vi "Periodic Tasks.vi"(8 "error in":errorcluster) -> ()   [LabVIEW 2012]
doc: "This VI runs in parallel to other tasks. It can contain as many user-defined periodic loops as you need. These can carry out PID or other sorts of timed response."
uses:
  climb_step_state.ctl
  <vilib>/Platform/TimedLoop/XDataNode/timing_clust.ctl
  <vilib>/Platform/TimedLoop/XDataNode/nitl_modes.ctl
  <vilib>/Platform/TimedLoop/XDataNode/wakeup.ctl
  <vilib>/Rock Robotics/WPI/Relay/WPI_RelayValue.ctl
  <vilib>/Rock Robotics/SystemInterfaces/Utilities/FPGA_UtilitiesLED Source.ctl
  <vilib>/Rock Robotics/SystemInterfaces/Utilities/FPGA_UtilitiesLED State.ctl
  Robot Global Data.vi
  <vilib>/Utility/file.llb/Read From Spreadsheet File (string).vi
  <vilib>/Rock Robotics/WPI/RobotDrive/WPI_RobotDriveGetSetRefNum.vi
  <vilib>/platform/TimedLoop/XDataNode/XDataNode.xnode
  <vilib>/Rock Robotics/WPI/Solenoid/WPI_SolenoidSetEnum.vi
  <vilib>/Rock Robotics/WPI/Solenoid/WPI_SolenoidValue.ctl
  <vilib>/Platform/TimedLoop/XDataNode/XDNodeRunTimeDep.lvlib
panel:
  in  "Reset 2":bool
  out "# elements in queue 3":i32
  in  "Reset":bool
  in  "Hold":bool=TRUE
  out "gear":i32
  out "arrived":bool
  in  "Set Point":dbl(slide)=1300.0 scale=-2000.0..1800.0
  in  "Velocity Profile":dbl[][](array[numeric])=[[400.0, 0.23, 0.1], [1000.0, 0.5, 0.1], [0.0, 0.8, 0.2]]
  out "motor":cluster{"Motor":dbl, "gear":i32}(graph)
  out "val":dbl
  out "Rate":cluster{"Rate":dbl, "Distance":dbl}(graph)
  in  "enc ms to wait":u32=100
  in  "Break Engaged 2":i32=120
  in  "Motor Run Time 2":dbl=0.4
  in  "Motor Pwr 2":dbl=-0.1
  in  "Break Disengaged 2":i32
  in  "Delay for disengage 2":dbl=0.2
  out "Enum 2":enum16{"Engaged", "Untension", "Disengaged"}(ring)
  out "Distance 2":dbl
  in  "Output 2":dbl(knob) scale=-1.0..1.0
  in  "Distance desired to\nretract tail hook completely 3":dbl
  in  "Current sensor load 3":dbl
  in  "Distance desired to \nretract (enough to detect if\nwe have weight on current sensor\nin next case) 3":dbl
  in  "distance to extend 3":dbl=850.0
  in  "half extend distance 2":dbl
  out "Rung counter 3":i32
  out "Climb Started? 2":bool
  in  "distance to flip 2":dbl=-600.0
  in  "Auto Flip Speed 2":dbl=-0.18
  out "Climb mode 2":enum16{"Wait", "Automatic", "Manual", "Abort"}(ring)
  out "Climb Step 2":T1
  in  "Climb Extend Tail Speed 2":dbl=1.0
  in  "Climb Retract Tail Speed 2":dbl=-0.9
  in  "Man Flip Speed 2":dbl=-0.75
  out "Turret Home Adjust 2":dbl
  in  "Sky Home Position 2":dbl
  out "Disciplined Sky Enc 2":dbl
  out "Sky Enc 2":dbl
  in  "Slow Retract 2":dbl=-0.25
  in  "Slow Extend 2":dbl=0.25
  in  "Robot Detect":T2(radio)
  out "Robot Detect":i32
  out "MAC Address":string
  out "Personality":string
  in  "Tab Control":T3(tab)
  out "FIFO":u32(graph)
  out "Shot Profile":dbl(graph)=3763.879304936955
  in  "Count":i32=80
  out "RPM @ Shot":dbl
  out "% err":dbl
  in  "Fire Log Enable":bool=TRUE
  in  "loop period (ms)":u32=200
  out "iterations":i32
  out "FIFO elements":u32
  in  "Burst":i32=75
  out "Save":bool
  out "Left Wheel Encoder":dbl
  out "Right Wheel Encoder":dbl
  out "LStopped":bool
  out "RStopped":bool
  out "Motor":dbl(graph)
  in  "Position":dbl(knob) scale=0.0..1500.0
  in  "SkyHook":dbl(knob) scale=-1.0..1.0
  out "Distance":dbl
  out "Home":bool
  in  "Motor Coerce":dbl=0.9
  in  "Lo Limit":dbl
  in  "Hi Limit":dbl=1500.0
  out "At Lo":bool
  out "At Hi":bool
  in  "Near Limit":dbl=200.0
  in  "Speed near Lim Up":dbl=0.2
  in  "Period":i64=51
  in  "Speed near Lim Dn":dbl=0.1
  in  "PID":bool
  in  "P":dbl(knob) scale=0.0..0.01
  out "err":dbl
  out "Rate":dbl
  in  "Auto Pitch":bool=TRUE
  in  "Elev Stable Tol (sec)":dbl(knob)=0.5044674819294696 scale=0.0..1.0
  out "Q 2":i32(graph)
  out "Current":dbl(graph)
  in  "A / V":dbl=13.66
  in  "Sample (s)":dbl=0.1
  in  "Log Enable":bool
  out "# elements in queue 2":i32
  out "Compressor Running":bool
  out "Right Odometer":dbl
  out "Left Odometer":dbl
  in  "Sample Rate (sec)":dbl=0.5
  in  "Sample?":bool=TRUE
  in  "Sample Rate (sec) 2":dbl=0.1
  in  "General Log Enable":bool=TRUE
  out "# elements in queue":i32
  in  "Gyro Gain (VoltsPerDegree/Second)":dbl(knob)=0.006611706614844206 scale=0.0..0.01
  out "Angle":dbl
  out "CornerShot Pitch":dbl
  out "Tow3 Offset Pitch":dbl
  out "Tow3 Offset RPM":dbl
  out "Tow1 Offset RPM":dbl
  out "Tow2 Offset RPM":dbl
  out "Tow1 Offset Pitch":dbl
  out "Tow2 Offset Pitch":dbl
  out "Std RPM":dbl
  out "Std Pitch":dbl
  out "Auton RPM":dbl
  out "Auton Pitch":dbl
  out "Wing RPM":dbl
  out "Wing Pitch":dbl
  out "Parameter Read":i32
  out "Tow1 Offset RPM 2":dbl
  out "Tow1 Offset Pitch 2":dbl
  out "Tow2 Offset RPM 2":dbl
  out "Tow2 Offset Pitch 2":dbl
  out "Tow3 Offset RPM 2":dbl
  out "Tow3 Offset Pitch 2":dbl
  out "QC iter":i32
  out "FIFO Elements":u32(graph)
  in  "loop period (ms) 2":u32=200
  out "Save Ascent":bool
  in  "Auto Ascent Log Enable":bool
  # "TDMS"
  # "TDMS"
  # "TDMS"
  # "TDMS"
  # "Range"
  # "Rate"
  # "Accel"
  # "Fire Cntrl Loop"
  # "Fire Cntrl Logging Loop"
  # "Sensor sensitivity is 73.20 mV / Amp"
  # "which is: 13.66 Amps / Volt"
  # "TDMS"
  # "Off will Disable\nOn will Sample at Rate"
  # "TDMS"
  # "On will sample at Rate\nOff will Disable"
  # "Positive Angles result from CW turns\nlooking down on Robot"
  # "Pos values back up\nNeg values go forward"
  # "Tower Shots"
  # "Auto Ascent Log"
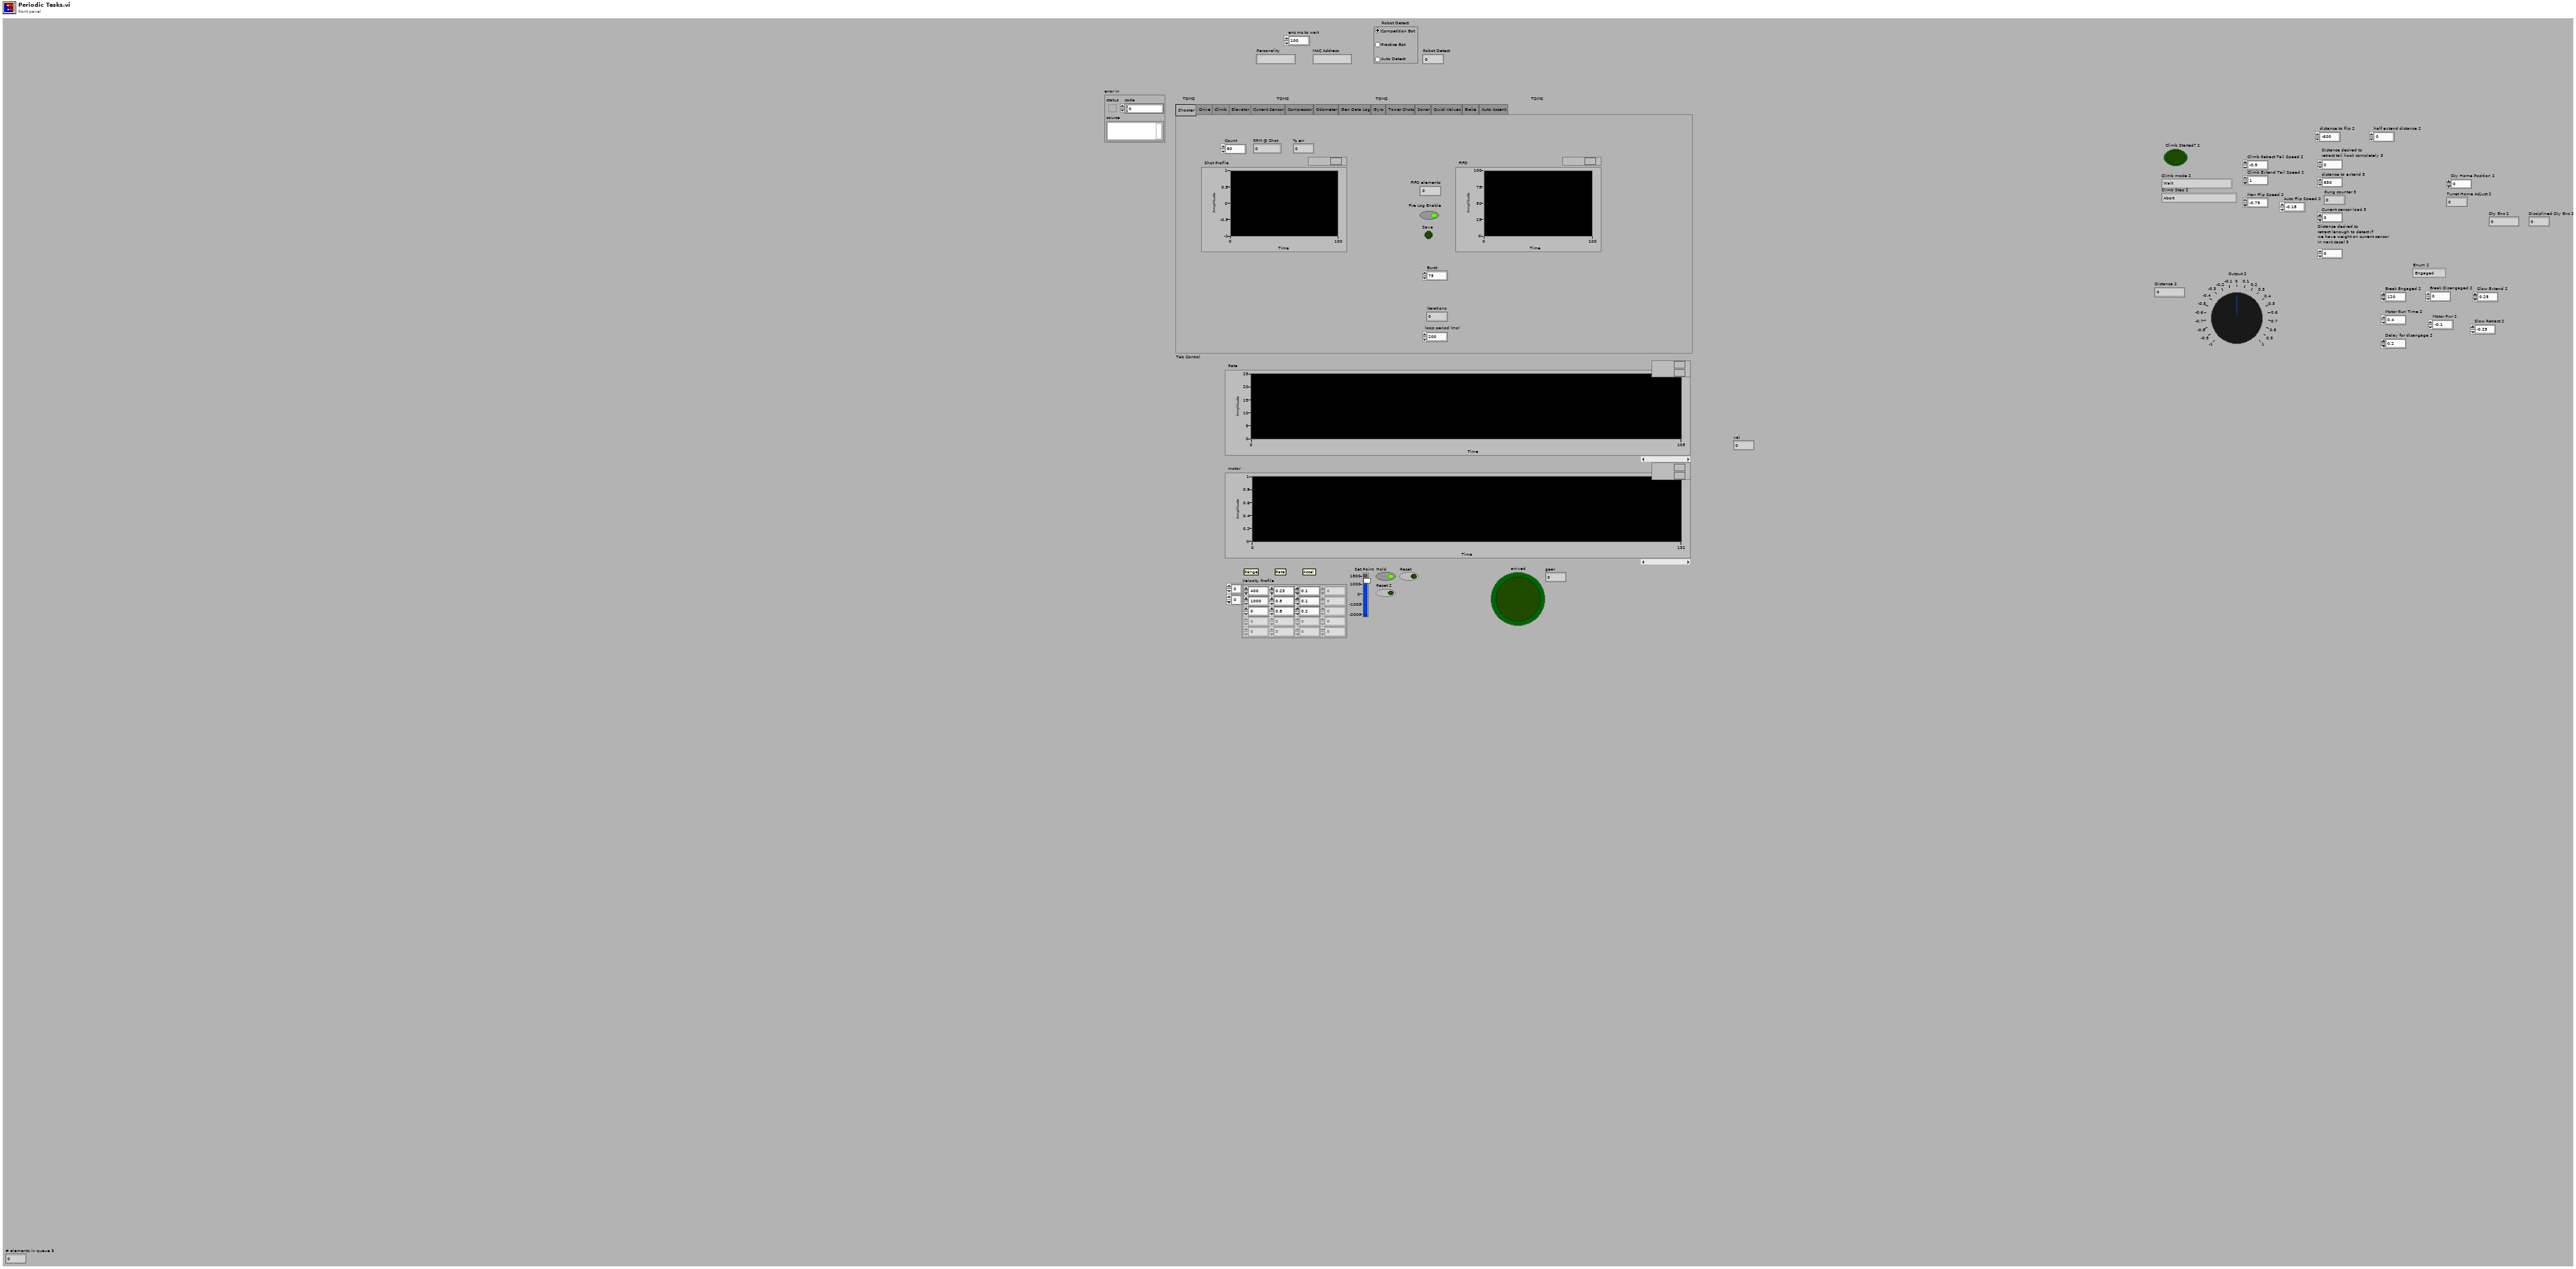
[diagram p1: front panel]
types:
  T1 = typedef "climb_step_state.ctl" = enum16{"Abort", "Approach Bar", "Approach +", "Climb Step 1", "Climb Step 2", "Climb Step 3", "Climb Step 4", "Climb Step 5", "Climb Step 6", "Climb Step 7", "Check Finished", "Check Continue"}
  T2 = enum32{"Competition Bot", "Practice Bot", "Auto Detect"}
  T3 = enum32{"Shooter", "Drive", "Climb", "Elevator", "Current Sensor", "Compressor", "Odometer", "Gen Data Log", "Gyro", "Tower Shots", "Sonar", "Quick Values", "Brake", "Auto Ascent"}
  T4 = enum16{"open", "open or create", "create or replace", "create", "open (read-only)"}
  T5 = cluster{"Driver Station Digital Input (1-8)[0]":bool, "Driver Station Digital Input (1-8)[1]":bool, "Driver Station Digital Input (1-8)[2]":bool, "Driver Station Digital Input (1-8)[3]":bool, "Driver Station Digital Input (1-8)[4]":bool, "Driver Station Digital Input (1-8)[5]":bool, "Driver Station Digital Input (1-8)[6]":bool, "Driver Station Digital Input (1-8)[7]":bool, "Driver Station Digital Input (1-8)[8]":bool}
  T6 = typedef "WPI_CounterDevRef.ctl" = cluster{"DevStatus":errorcluster, "CntIndex":T7}
  T7 = typedef "FPGA_CounterCtrSystemIndex.ctl" = enum8{"Ctr 0", "Ctr 1", "Ctr 2", "Ctr 3", "Ctr 4", "Ctr 5", "Ctr 6", "Ctr 7", "Invalid"}
  T8 = typedef "WPI_MotorControlDeviceRef.ctl" = cluster{"DeviceStatus":errorcluster, "Type":enum16{"PWM", "CAN"}, "PWM":cluster{"Digital Module":T9, "PWM Channel":T10, "DeadBand":T11}, "CAN":cluster{"Device Number":u8, "Control Mode":T12, "Semaphore":T13, "Max Vout":dbl}, "Invert":bool, "TransformRef":T14, "InvTransformRef":T14}
  T9 = typedef "FPGA_TypedefDigitalModule.ctl" = enum16{"Digital Module 1", "Digital Module 2"}
  T10 = typedef "FPGA_DIOPWMChannel.ctl" = enum8{"PWM 1", "PWM 2", "PWM 3", "PWM 4", "PWM 5", "PWM 6", "PWM 7", "PWM 8", "PWM 9", "PWM 10", "Invalid"}
  T11 = typedef "WPI_PWMDeadband.ctl" = cluster{"Name":string, "maxPositivePwm":i32, "minPositivePwm":i32, "centerPwm":i32, "maxNegativePwm":i32, "minNegativePwm":i32, "angularRange":u16}
  T12 = typedef "WPI_CANJaguar_ControlMode.ctl" = enum8{"Percent VBus", "Current", "Speed", "Position", "Voltage"}
  T13 = typedef "Semaphore RefNum" = refnum<k1>
  T14 = typedef "WPI_PWMTransform_ConPane.ctl" = refnum<vi>
  T15 = typedef "WPI_GyroDevRef.ctl" = cluster{"DevStatus":errorcluster, "Analog Module":T16, "Analog Channel":T17, "Offset":dbl, "Gain (VoltsPerDegree/Second)":dbl}
  T16 = typedef "FPGA_TypedefAnalogModule.ctl" = enum16{"Analog Module 1", "Analog Module 2"}
  T17 = typedef "FPGA_AIChannel.ctl" = enum8{"AI 1", "AI 2", "AI 3", "AI 4", "AI 5", "AI 6", "AI 7", "AI 8", "Invalid"}
  T18 = typedef "WPI_EncoderDevRef.ctl" = cluster{"DevStatus":errorcluster, "EncoderIndex":T19, "CounterIndex":T7, "DistancePerCount":dbl, "Decoding Type":T20}
  T19 = typedef "FPGA_EncoderIdx.ctl" = enum8{"Enc 0", "Enc 1", "Enc 2", "Enc 3", "Invalid"}
  T20 = typedef "WPI_EncoderType.ctl" = enum16{"1x", "2x", "4x"}
  T21 = typedef "WPI_SolenoidDevRef.ctl" = cluster{"DevStatus":errorcluster, "Solenoid Module":T22, "Forward Solenoid Channel":T23, "Reverse Solenoid Channel":T23}
  T22 = typedef "FPGA_TypedefSolenoidModule.ctl" = enum16{"Solenoid Module 1", "Solenoid Module 2"}
  T23 = typedef "WPI_SolenoidChannel.ctl" = enum8{"Solenoid 1", "Solenoid 2", "Solenoid 3", "Solenoid 4", "Solenoid 5", "Solenoid 6", "Solenoid 7", "Solenoid 8", "Invalid"}
  T24 = typedef "WPI_RelayDevRef.ctl" = cluster{"DevStatus":errorcluster, "Relay Channel":T25, "Digital Module":T9, "Relay Direction":T26}
  T25 = typedef "FPGA_DIORelayChannel.ctl" = enum8{"Relay 1", "Relay 2", "Relay 3", "Relay 4", "Relay 5", "Relay 6", "Relay 7", "Relay 8", "Invalid"}
  T26 = typedef "WPI_RelayDirection.ctl" = enum16{"Both directions", "Forward only", "Reverse only"}
  T27 = typedef "WPI_DigitalInputDevRef.ctl" = cluster{"DevStatus":errorcluster, "DIO Channel":T28, "Digital Module":T9}
  T28 = typedef "FPGA_DIOChannel.ctl" = enum8{"DIO 1", "DIO 2", "DIO 3", "DIO 4", "DIO 5", "DIO 6", "DIO 7", "DIO 8", "DIO 9", "DIO 10", "DIO 11", "DIO 12", "DIO 13", "DIO 14", "Invalid"}
  T29 = typedef "XDNodeRunTimeDep.lvlib/timing_clust.ctl" = cluster{"Expected End [f-1]":u64, "Actual End [f-1]":u64, "Finished Late? [f-1]":bool, "Expected End [i-1]":u64, "Actual End [i-1]":u64, "Finished Late? [i-1]":bool, "Expected Start [i]":u64, "Actual Start [i]":u64, "Expected Start [f]":u64, "Actual Start [f]":u64, "Source Name":string, "Structure Name":string, "Period":i64, "Deadline":i64, "Offset":i64, "Start":i64, "Priority":i32, "Timeout":i32, "Mode":T30, "Wakeup Reason":T31, "Error":errorcluster, "Source Type":string, "Secondary Source Type":string, "Global End Time":u64, "Global Start Time":u64, "Frame Duration":u64, "Iteration Duration":u64, "Assigned CPU":i32, "I/O Scan Engine Mode":u32}
  T30 = typedef "XDNodeRunTimeDep.lvlib/nitl_modes.ctl" = enum32{"No Change", "Process missed periods, maintain original phase", "Discard missed periods, maintain original phase", "Process missed periods, ignore original phase", "Discard missed periods, ignore original phase"}
  T31 = typedef "XDNodeRunTimeDep.lvlib/wakeup.ctl" = enum32{"Normal", "Aborted", "Asynchronous wakeup", "Timing source error", "Timed loop error", "Timeout"}
  T32 = typedef "WPI_AnalogChannelDevRef.ctl" = cluster{"DevStatus":errorcluster, "Analog Module":T16, "Analog Channel":T17}
  T33 = typedef "FPGA_UtilitiesLED State.ctl" = enum16{"Off", "On", "Toggle"}
  T34 = typedef "FPGA_UtilitiesLED Source.ctl" = enum16{"User LED", "FPGA LED"}
  T35 = cluster{"all rows[0]":string, "all rows[1]":string, "all rows[2]":string, "all rows[3]":string, "all rows[4]":string, "all rows[5]":string, "all rows[6]":string, "all rows[7]":string, "all rows[8]":string}
  T36 = typedef "fire_step_state.ctl" = enum16{"static", "manual", "saftey_down", "saftey_up", "check_saftey", "fire"}
  T37 = typedef "WPI_RelayValue.ctl" = enum16{"Off", "On", "Forward", "Reverse"}
  T38 = typedef "WPI_ServoDeviceRef.ctl" = cluster{"DeviceStatus":errorcluster, "Digital Module":T9, "PWM Channel":T10, "DeadBand":T11}
  T39 = typedef "WPI_RobotDriveDevRef.ctl" = cluster{"DevStatus":errorcluster, "Motors[]":T8[], "Square Inputs":bool, "Max Output":dbl, "Isochronous":bool}
  T40 = typedef "WPI_SolenoidValue.ctl" = enum16{"Off", "On", "Forward", "Reverse"}
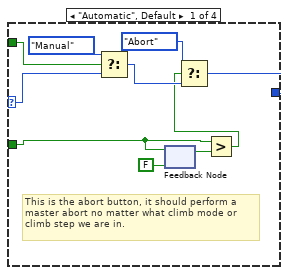
[diagram p2: hidden frame]
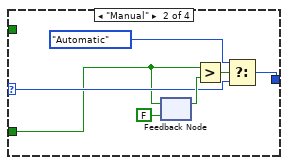
[diagram p3: hidden frame]
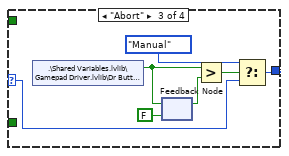
[diagram p4: hidden frame]
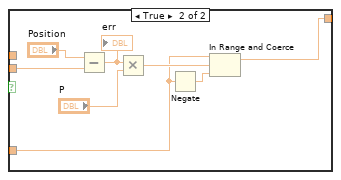
[diagram p5: hidden frame]
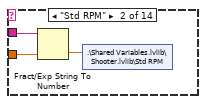
[diagram p20: hidden frame]
diagram:
  w6 = 5 ("dimension size")
  w13 = climb_step_state."Approach Bar" ("Climb Step")
  w65 = path "C:/tmp/Odometer.tdms" ("file path (dialog if empty)")
  (unwired) "NI_DiskCacheSize"
  w114 = 18 ("dimension size")
  (unwired) "This code flashes the USER1 LED on the cRIO.  It is a simple way to let you know your code is running on the cRIO.  You can leave this code if you find it helpful, or delete it if you don't want it."
  (unwired) "This VI is a good place to take care of periodic tasks such as control loops.\n\nAdd code to the existing loops, or duplicate a loop to define a new rate. You can allocate I/O references here, or in Begin.vi.\n\nPeriodic loops will often operate with setpoints from other loops. Use a global variable such as Robot Global Data for sharing data between loops."
  # "Auto Ascent FIFO Setup"
  # "Size of Auto Ascent Log"
  # "Periodic Data FIFO Setup"
  # "Odometer"
  # "Size of Fire Cntrl Log"
  # "Pre-Allocate Array to improve \nDeterminism when Data Logging"
  # "Removed Safety Servo and States\nBatWings\nDisc Drive is full time\nRemoved Override\nRemoved Drive stopped\nRemoved settings for other shooter\nTrimmed Log entries"
  # "Data Log Enable"
  # "Periodic Data Log Setup"
  n1 = while {
    stop <- FALSE stop-if-true
    n2 = call <vilib>:"WPI_DriverStationGet Digital Input.vi"() -> ("Driver Station Digital Input (1-8)"=w136:bool[])  [unwired: 11 in]
    n3 = Array To Cluster(array=w136) -> (cluster=w135:T5)
    n4 = Unbundle By Name(w135) -> ("Driver Station Digital Input (1-8)[7]"=w134:bool)
    n5 = Wait (ms)(milliseconds to wait=u32 500) -> ()  [unwired: 1 out]
    n6 = shared-variable ".\\Shared Variables.lvlib\\System.lvlib\\Data Log"(w134) -> ()  [unwired: 1 in, 1 out]
  }
  n7 = Get Date/Time In Seconds() -> (seconds since 1Jan1904=w124:timestamp)
  n8 = Format Date/Time String(time format string (%c)="%m-%#d-%Y %H%M", seconds (now)=w124, UTC format=FALSE) -> (date/time string=w129:string)
  n9 = Concatenate Strings("PeriodicDataLog" ("string"), w129, ".tdms" ("string")) -> (w131:string)
  n10 = Build Path(base path=path "C:/tmp" ("file path (dialog if empty)"), name or relative path=w131) -> (appended path=w111:path)
  n11 = TDMS Open(6:TRUE ("disable buffering? (T)"), 7:enum16{"1.0", "2.0"}."2.0" ("file format version (2.0)"), 10:T4."open or create" ("operation (0:open)"), 11:w111) -> (3:w93:refnum<k34>)  [unwired: 2 in, 1 out]
  n12 = for {
    N: 18 -> [_]
    tunnel: string[] ["Time", "Iteration", "Mode", "Raw Prime", "Cultured Prime", "Raw On Deck", "Cultured On Deck", "Button 6 Op (Fire)", "Fire Case", "RPM", "Elevator", "Shooter Bump", "Elevator Bump", "Button 2 Op (Wish)", "Shooter Stable", "Indexer", "Air Lock", "FIFO Buffer", "", "", "", "", "", "", "", "", ""] ("channel name(s) in (Untitled)") -> [w144] mode=indexing
    tunnel: "Fire Control" ("group name in (Untitled)") -> [w143]
    tunnel: w93 -> [w142]
    tunnel: [w141] -> w34
    tunnel: "NI_MimimumBufferSize" -> [w140]
    tunnel: 1000 -> [w139]
    n13 = TDMS Set Properties(5:w139, 7:w140, 9:w144, 10:w143, 11:w142) -> (3:w141:refnum<k34>)  [unwired: 1 in, 3 out]
  }
  n14 = Initialize Array(0 ("element"), w6) -> (w18:i32[])
  n15 = Initialize Array(0 ("element"), w114) -> (w112:i32[])
  n16 = To Unsigned Long Integer(number=w6) -> (unsigned 32bit integer=w5:u32)
  n17 = To Unsigned Long Integer(number=w114) -> (unsigned 32bit integer=w113:u32)
  n18 = RT FIFO Create(0:"Auto Ascent FIFO" ("name (unnamed)"), 1:w18, 4:u32 100 ("size (10)"), 6:w5) -> (8:w19:refnum<k33>)  [unwired: 4 in, 2 out]
  n19 = RT FIFO Create(0:"Fire Control FIFO" ("name (unnamed)"), 1:w112, 4:u32 100 ("size (10)"), 6:w113) -> (8:w116:refnum<k33>)  [unwired: 4 in, 2 out]
  n20 = call "cRIO MAC.vi"() -> ("MAC Address"=→"MAC Address":string, "Personality"=w96:string)  [unwired: 2 in]
  "Personality" <- w96
  n21 = call <vilib>:"WPI_CounterRefNum Registry Get.vi"("refnum name"="shooterRpm") -> ("CounterDevRef"=w86:T6)  [unwired: 9 in, 1 out]
  n22 = call <vilib>:"WPI_MotorControlRefNum Registry Get.vi"("refnum name"="shooterThrust") -> ("MotorControlDevRef"=w84:T8)  [unwired: 9 in, 1 out]
  n23 = disable-structure shown="Disabled" {
    disable-tunnel: w65 -> [w145 _]
    frame Disabled {
      n24 = TDMS Defragment(7:w145) -> ()  [unwired: 1 in, 1 out]
    }
    frame Enabled {
    }
  }
  n25 = Get Date/Time In Seconds() -> (seconds since 1Jan1904=w56:timestamp)
  n26 = Initialize Array(0.0 ("element"), 3 ("dimension size")) -> (w47:dbl[])
  n27 = call <vilib>:"WPI_GyroRefNum Registry Get.vi"("refnum name"="turnGyro") -> ("GyroDevRef"=w70:T15)  [unwired: 9 in, 1 out]
  n28 = TDMS Open(7:enum16{"1.0", "2.0"}."2.0" ("file format version (2.0)"), 10:T4."open or create" ("operation (0:open)"), 11:w65) -> (3:w33:refnum<k34>)  [unwired: 3 in, 1 out]
  n29 = call <vilib>:"WPI_EncoderRefNum Registry Get.vi"("refnum name"="leftWheelEncoder") -> ("EncoderDevRef"=w74:T18)  [unwired: 9 in, 1 out]
  n30 = call <vilib>:"WPI_EncoderRefNum Registry Get.vi"("refnum name"="rightWheelEncoder") -> ("EncoderDevRef"=w73:T18)  [unwired: 9 in, 1 out]
  n31 = Initialize Array(0.0 ("element"), 4 ("dimension size")) -> (w39:dbl[])
  n32 = call <vilib>:"WPI_SolenoidRefNum Registry Get.vi"("refnum name"="discSolenoid") -> ("SolenoidDevRef"=w101:T21)  [unwired: 9 in, 1 out]
  n33 = call <vilib>:"WPI_RelayRefNum Registry Get.vi"("refnum name"="conveyor") -> ("RelayDevRef"=w99:T24)  [unwired: 9 in, 1 out]
  n34 = call <vilib>:"WPI_SolenoidRefNum Registry Get.vi"("refnum name"="fireSolenoid") -> ("SolenoidDevRef"=w100:T21)  [unwired: 9 in, 1 out]
  n35 = call <vilib>:"WPI_DigitalInputRefNum Registry Get.vi"("refnum name"="breakBeamOnDeck") -> ("DigitalInputDevRef"=w102:T27)  [unwired: 9 in, 1 out]
  n36 = call <vilib>:"WPI_DigitalInputRefNum Registry Get.vi"("refnum name"="breakBeamPrime") -> ("DigitalInputDevRef"=w103:T27)  [unwired: 9 in, 1 out]
  n37 = To Double Precision Float(number=w56) -> (double precision float=w55:dbl)
  n38 = call <vilib>:"WPI_DigitalInputRefNum Registry Get.vi"("refnum name"="compressorSwitch") -> ("DigitalInputDevRef"=w132:T27)  [unwired: 9 in, 1 out]
  n39 = node-c288(i64 51 ("Period")) -> (w30:T29)  [unwired: 3 in]
  n40 = node-c288(i64 16 ("Period")) -> (w110:T29)  [unwired: 3 in]
  n41 = node-c288(i64 11 ("Period")) -> (w89:T29)  [unwired: 3 in]
  n42 = Get Date/Time In Seconds() -> (seconds since 1Jan1904=w44:timestamp)
  n43 = Get Date/Time In Seconds() -> (seconds since 1Jan1904=w52:timestamp)
  n44 = Obtain Queue(max queue size (-1, unlimited)=100, name (unnamed)="Q", element data type=w47) -> (queue out=w46:refnum<queue>)  [unwired: 2 in, 2 out]
  n45 = Obtain Queue(max queue size (-1, unlimited)=100, name (unnamed)="Q2", element data type=w39) -> (queue out=w38:refnum<queue>)  [unwired: 2 in, 2 out]
  n46 = call <vilib>:"WPI_AnalogChannelRefNum Registry Get.vi"("refnum name"="climbMotorCurrent") -> ("AIDeviceRef"=w35:T32)  [unwired: 9 in, 1 out]
  n47 = To Double Precision Float(number=w44) -> (double precision float=w43:dbl)
  n48 = To Double Precision Float(number=w52) -> (double precision float=w51:dbl)
  n49 = while {
    stop <- FALSE stop-if-true
    # "This global is written to in the Autonomous and Teleop VIs"
    # "Flash the USER1 LED with the rate controlled from Autonomous and Teleop"
    n50 = global read "Robot Global Data.vi" "LED toggle rate (ms)"() -> (w146:u32)
    n51 = call <vilib>:"WPI_UtilitiesFRC LEDs.vi"("State"=FPGA_UtilitiesLED_State."Toggle", "LED Type"=FPGA_UtilitiesLED_Source."User LED") -> ()  [unwired: 1 in, 9 out]
    n52 = Wait (ms)(milliseconds to wait=w146) -> ()  [unwired: 1 out]
  }
  n53 = while "Robot Detect Loop" {
    tunnel: w96 -> [w152]
    tunnel: [w150] -> w119
    i -> [w153]
    stop <- w156 stop-if-true
    # "Auto-Detect"
    n54 = Equal?(x="Robot Detect", y=T2."Competition Bot") -> (x = y?=w158:bool)
    n55 = Equal?(x="Robot Detect", y=T2."Practice Bot") -> (x = y?=w157:bool)
    n56 = Select(t="Pract Bot - Friz 1", s=w157, f=w152) -> (s? t:f=w159:string)
    n57 = Not Equal?(x=w152, y="") -> (x != y?=w154:bool)
    n58 = Select(t="Comp Bot - Friz 2", s=w158, f=w159) -> (s? t:f=w150:string)
    n59 = global write "Robot Global Data.vi" "Personality"(w150) -> ()
    n60 = Compound Arithmetic op=OR(w158, w157, w154) -> (w156:bool)
    n61 = Wait (ms)(milliseconds to wait=u32 30) -> ()  [unwired: 1 out]
    "Robot Detect" <- w153
  }
  n62 = while "Quick-change parameters" {
    tunnel: [w165] -> w95
    stop <- w165 stop-if-true
    w165 = TRUE
    n63 = call-poly <vilib>:"Read From Spreadsheet File.vi"("delimiter (\\t)"="=" ("delimiter (\\t)"), "file path (dialog if empty)"=path "C:/tmp/2013 Code Parameters.csv" ("datalog path (use dialog)")) -> ("all rows"=w166:string[][])  [unwired: 5 in, 4 out]
    n64 = for {
      tunnel: w166 -> [w174] mode=indexing
      i -> [w169]
      n65 = Array To Cluster(array=w174) -> (cluster=w173:T35)
      n66 = Unbundle By Name(w173) -> ("all rows[0]"=w172:string, "all rows[1]"=w171:string)
      n67 = case shown="\"Auton RPM\"" w172 {
        tunnel: w171 -> [_ w177 w180 w183 w186 w189 w192 w195 w198 w201 w204 w207 w210 w213]
        tunnel: 0.0 -> [_ w176 w179 w182 w185 w188 w191 w194 w197 w200 w203 w206 w209 w212]
        frame "", Default {
        }
        frame "Std RPM" {
          n68 = Fract/Exp String To Number(string=w177, default (0 dbl)=w176) -> (number=w175:dbl)  [unwired: 2 in, 1 out]
          n69 = shared-variable ".\\Shared Variables.lvlib\\Shooter.lvlib\\Std RPM"(w175) -> ()  [unwired: 1 in, 1 out]
        }
        frame "Std Pitch" {
          n70 = Fract/Exp String To Number(string=w180, default (0 dbl)=w179) -> (number=w178:dbl)  [unwired: 2 in, 1 out]
          n71 = shared-variable ".\\Shared Variables.lvlib\\Elevator.lvlib\\Std Pitch"(w178) -> ()  [unwired: 1 in, 1 out]
        }
        frame "Auton RPM" {
          n72 = Fract/Exp String To Number(string=w183, default (0 dbl)=w182) -> (number=w181:dbl)  [unwired: 2 in, 1 out]
          n73 = shared-variable ".\\Shared Variables.lvlib\\Shooter.lvlib\\Auton RPM"(w181) -> ()  [unwired: 1 in, 1 out]
        }
        frame "Auton Pitch" {
          n74 = Fract/Exp String To Number(string=w186, default (0 dbl)=w185) -> (number=w184:dbl)  [unwired: 2 in, 1 out]
          n75 = shared-variable ".\\Shared Variables.lvlib\\Elevator.lvlib\\Auton Pitch"(w184) -> ()  [unwired: 1 in, 1 out]
        }
        frame "Wing RPM" {
          n76 = Fract/Exp String To Number(string=w189, default (0 dbl)=w188) -> (number=w187:dbl)  [unwired: 2 in, 1 out]
          n77 = shared-variable ".\\Shared Variables.lvlib\\Shooter.lvlib\\Wing RPM"(w187) -> ()  [unwired: 1 in, 1 out]
        }
        frame "Wing Pitch" {
          n78 = Fract/Exp String To Number(string=w192, default (0 dbl)=w191) -> (number=w190:dbl)  [unwired: 2 in, 1 out]
          n79 = shared-variable ".\\Shared Variables.lvlib\\Elevator.lvlib\\Wing Pitch"(w190) -> ()  [unwired: 1 in, 1 out]
        }
        frame "Tow1 Offset RPM" {
          n80 = Fract/Exp String To Number(string=w195, default (0 dbl)=w194) -> (number=w193:dbl)  [unwired: 2 in, 1 out]
          "Tow1 Offset RPM" <- w193
          n81 = shared-variable ".\\Shared Variables.lvlib\\Shooter.lvlib\\Tow1 Offset RPM"(w193) -> ()  [unwired: 1 in, 1 out]
        }
        frame "Tow1 Offset Pitch" {
          n82 = Fract/Exp String To Number(string=w198, default (0 dbl)=w197) -> (number=w196:dbl)  [unwired: 2 in, 1 out]
          "Tow1 Offset Pitch" <- w196
          n83 = shared-variable ".\\Shared Variables.lvlib\\Elevator.lvlib\\Tow1 Offset Pitch"(w196) -> ()  [unwired: 1 in, 1 out]
        }
        frame "Tow2 Offset RPM" {
          n84 = Fract/Exp String To Number(string=w201, default (0 dbl)=w200) -> (number=w199:dbl)  [unwired: 2 in, 1 out]
          "Tow2 Offset RPM" <- w199
          n85 = shared-variable ".\\Shared Variables.lvlib\\Shooter.lvlib\\Tow2 Offset RPM"(w199) -> ()  [unwired: 1 in, 1 out]
        }
        frame "Tow2 Offset Pitch" {
          n86 = Fract/Exp String To Number(string=w204, default (0 dbl)=w203) -> (number=w202:dbl)  [unwired: 2 in, 1 out]
          "Tow2 Offset Pitch" <- w202
          n87 = shared-variable ".\\Shared Variables.lvlib\\Elevator.lvlib\\Tow2 Offset Pitch"(w202) -> ()  [unwired: 1 in, 1 out]
        }
        frame "Tow3 Offset RPM" {
          n88 = Fract/Exp String To Number(string=w207, default (0 dbl)=w206) -> (number=w205:dbl)  [unwired: 2 in, 1 out]
          "Tow3 Offset RPM" <- w205
          n89 = shared-variable ".\\Shared Variables.lvlib\\Shooter.lvlib\\Tow3 Offset RPM"(w205) -> ()  [unwired: 1 in, 1 out]
        }
        frame "Tow3 Offset Pitch" {
          n90 = Fract/Exp String To Number(string=w210, default (0 dbl)=w209) -> (number=w208:dbl)  [unwired: 2 in, 1 out]
          "Tow3 Offset Pitch" <- w208
          n91 = shared-variable ".\\Shared Variables.lvlib\\Elevator.lvlib\\Tow3 Offset Pitch"(w208) -> ()  [unwired: 1 in, 1 out]
        }
        frame "CornerShot Pitch" {
          n92 = Fract/Exp String To Number(string=w213, default (0 dbl)=w212) -> (number=w211:dbl)  [unwired: 2 in, 1 out]
          "CornerShot Pitch" <- w211
          n93 = shared-variable ".\\Shared Variables.lvlib\\Elevator.lvlib\\CornerShot Pitch"(w211) -> ()  [unwired: 1 in, 1 out]
        }
      }
      "QC iter" <- w169
    }
  }
  n94 = timed-loop "Fire Control Loop\nTime Critical" {
    tunnel: w103 -> [w218]
    tunnel: w102 -> [w247]
    tunnel: w101 -> [w246]
    tunnel: w100 -> [w245]
    tunnel: w99 -> [w244]
    tunnel: w112 -> [w219]
    timing: w110 -> [_]
    timing-out: [_] -> w109
    tunnel: w116 -> [w223]
    tunnel: w55 -> [w216]
    i -> [w217]
    stop <- FALSE stop-if-true
    w230 = 4200.0 ("x")
    n95 = feedback #1() -> (w225:T36)  [unwired: 1 in]
    n96 = call "Fire Control Loop.vi"("Prime BB DevRef"=w218, "OnDeck BB DevRef"=w247, "Fire Log Enable"="Fire Log Enable", "FireDevRef"=w245, "Time Ref"=w216, "ConveyorDevRef"=w244, "rt fifo"=w223, "Fire State In"=w225, "LogArray"=w219, "iteration"=w217, "IndexerDevRef"=w246) -> ("Fire"=w236:bool, "Fire State Out"=w226:T36, "# elements"=w222:u32)  [unwired: 2 in]
    "FIFO elements" <- w222
    "FIFO" <- w222
    n97 = feedback-in #1(w226) -> ()
    n98 = shared-variable ".\\Shared Variables.lvlib\\Shooter.lvlib\\Shooter RPM Response"() -> (w234:dbl)  [unwired: 1 in, 1 out]
    n99 = local read "Burst"() -> (w221:i32)
    n100 = Greater?(x=w222, y=w221) -> (0:→"Save":bool)
    n101 = feedback #2() -> (w235:bool)  [unwired: 1 in]
    n102 = feedback-in #2(w236) -> ()
    n103 = Greater?(x=w236, y=w235) -> (0:w233:bool)
    n104 = feedback #3(0) -> (w242:i32)
    n105 = Select(t=w217, s=w233, f=w242) -> (s? t:f=w241:i32)
    n106 = feedback-in #3(w241) -> ()
    n107 = feedback #4() -> (w237:dbl)  [unwired: 1 in]
    n108 = Select(t=w234, s=w233, f=w237) -> (s? t:f=w232:dbl)
    "RPM @ Shot" <- w232
    n109 = feedback-in #4(w232) -> ()
    n110 = Add(x=w241, y="Count") -> (x+y=w239:i32)
    n111 = Less Or Equal?(x=w217, y=w239) -> (x <= y?=w238:bool)
    n112 = case shown="True" w238 {
      tunnel: w234 -> [_ w248]
      frame False {
      }
      frame True {
        "Shot Profile" <- w248
      }
    }
    n113 = Subtract(x=w230, y=w232) -> (x-y=w231:dbl)
    n114 = Divide(x=w231, y=w230) -> (x/y=w229:dbl)
    n115 = Multiply(x=w229, y=100.0) -> (x*y=→"% err":dbl)
    n116 = call "Elapsed Times.vi"("Call Name"="F") -> ()  [unwired: 2 in, 1 out]
  }
  n117 = while "Quick-change File I/O Verification Display" {
    i -> [w274]
    stop <- w277 stop-if-true
    n118 = shared-variable ".\\Shared Variables.lvlib\\Shooter.lvlib\\Std RPM"() -> (→"Std RPM":dbl, error out=w261:errorcluster)  [unwired: 1 in]
    n119 = shared-variable ".\\Shared Variables.lvlib\\Elevator.lvlib\\Std Pitch"(error in=w261) -> (→"Std Pitch":dbl, error out=w260:errorcluster)
    n120 = shared-variable ".\\Shared Variables.lvlib\\Shooter.lvlib\\Auton RPM"(error in=w260) -> (→"Auton RPM":dbl, error out=w259:errorcluster)
    n121 = shared-variable ".\\Shared Variables.lvlib\\Elevator.lvlib\\Auton Pitch"(error in=w259) -> (→"Auton Pitch":dbl, error out=w258:errorcluster)
    n122 = shared-variable ".\\Shared Variables.lvlib\\Shooter.lvlib\\Wing RPM"(error in=w258) -> (→"Wing RPM":dbl, error out=w257:errorcluster)
    n123 = shared-variable ".\\Shared Variables.lvlib\\Elevator.lvlib\\Wing Pitch"(error in=w257) -> (→"Wing Pitch":dbl, error out=w256:errorcluster)
    n124 = shared-variable ".\\Shared Variables.lvlib\\Shooter.lvlib\\Tow1 Offset RPM"(error in=w256) -> (→"Tow1 Offset RPM 2":dbl, error out=w255:errorcluster)
    n125 = shared-variable ".\\Shared Variables.lvlib\\Elevator.lvlib\\Tow1 Offset Pitch"(error in=w255) -> (→"Tow1 Offset Pitch 2":dbl, error out=w254:errorcluster)
    n126 = shared-variable ".\\Shared Variables.lvlib\\Shooter.lvlib\\Tow2 Offset RPM"(error in=w254) -> (→"Tow2 Offset RPM 2":dbl, error out=w253:errorcluster)
    n127 = shared-variable ".\\Shared Variables.lvlib\\Elevator.lvlib\\Tow2 Offset Pitch"(error in=w253) -> (→"Tow2 Offset Pitch 2":dbl, error out=w252:errorcluster)
    n128 = shared-variable ".\\Shared Variables.lvlib\\Shooter.lvlib\\Tow3 Offset RPM"(error in=w252) -> (→"Tow3 Offset RPM 2":dbl, error out=w251:errorcluster)
    n129 = shared-variable ".\\Shared Variables.lvlib\\Elevator.lvlib\\Tow3 Offset Pitch"(error in=w251) -> (w266:dbl)  [unwired: 1 out]
    "Tow3 Offset Pitch 2" <- w266
    n130 = Not Equal?(x=w266, y=0.0) -> (x != y?=w277:bool)
    n131 = Wait (ms)(milliseconds to wait=u32 100) -> ()  [unwired: 1 out]
    "Parameter Read" <- w274
  }
  n132 = timed-loop "Shooter Control Loop\nTime Critical" {
    tunnel: w84 -> [w278]
    tunnel: w86 -> [w279]
    timing: w89 -> [_]
    timing-out: [_] -> w88
    stop <- FALSE stop-if-true
    n133 = call "Elapsed Times.vi"("Call Name"="Shoot") -> ()  [unwired: 2 in, 1 out]
    n134 = call "Shooter Loop.vi"("MotorControlDevRef"=w278, "CounterDevRef"=w279) -> ()  [unwired: 1 in]
  }
  n135 = while "Auto Ascent Logging Loop" {
    tunnel: w19 -> [w291]
    tunnel: w18 -> [w290]
    tunnel: w34 -> [w289]
    stop <- FALSE stop-if-true
    n136 = local read "Save Ascent"() -> (w287:bool)
    n137 = call "Elapsed Times.vi"("Call Name"="AA Log") -> ()  [unwired: 2 in, 1 out]
    n138 = local read "Burst"() -> (w284:i32)
    n139 = call "Auto Ascent Data Logger.vi"("Save"=w287, "Init Array"=w290, "Burst"=w284, "rt fifo"=w291, "TDMS Refnum"=w289) -> ()  [unwired: 7 in]
    n140 = Wait (ms)(milliseconds to wait="loop period (ms) 2") -> ()  [unwired: 1 out]
  }
  n141 = while "General Data Logging Loop" {
    tunnel: w34 -> [w300]
    tunnel: w51 -> [w299]
    tunnel: w47 -> [w294]
    tunnel: w46 -> [w293]
    stop <- FALSE stop-if-true
    n142 = shared-variable ".\\Shared Variables.lvlib\\System.lvlib\\Data Log"() -> (w295:bool)  [unwired: 1 in, 1 out]
    n143 = And(x="General Log Enable", y=w295) -> (x .and. y?=w297:bool)
    n144 = case shown="True" w297 {
      tunnel: w300 -> [_ w306]
      tunnel: w299 -> [_ w310]
      tunnel: w294 -> [_ w307]
      tunnel: w293 -> [_ w305]
      frame False {
        # "Logging is disabled"
      }
      frame True {
        w301 = 50 ("y")
        n145 = Get Date/Time In Seconds() -> (seconds since 1Jan1904=w314:timestamp)
        n146 = Get Queue Status(queue=w305) -> (queue out=w304:refnum<queue>, # elements in queue=w303:i32)  [unwired: 2 in, 6 out]
        "# elements in queue" <- w303
        n147 = To Double Precision Float(number=w314) -> (double precision float=w313:dbl)
        n148 = Greater Or Equal?(x=w303, y=w301) -> (x >= y?=w302:bool)
        n149 = Subtract(x=w313, y=w310) -> (x-y=w309:dbl)
        n150 = Quotient & Remainder(x=w309, y="Sample Rate (sec) 2") -> (floor(x/y)=w311:dbl)  [unwired: 1 out]
        n151 = feedback #5() -> (w312:dbl)  [unwired: 1 in]
        n152 = feedback-in #5(w311) -> ()
        n153 = Greater?(x=w311, y=w312) -> (0:w308:bool)
        n154 = case shown="True" w308 {
          tunnel: w309 -> [_ w329]
          tunnel: w307 -> [_ w330]
          tunnel: w305 -> [_ w326]
          frame False {
            # "Logging to Queue is Off during not-sample time period"
          }
          frame True {
            # "Queue up data at Sample time"
            n155 = shared-variable ".\\Shared Variables.lvlib\\Shooter.lvlib\\Shooter RPM Response"() -> (w328:dbl, error out=w334:errorcluster)  [unwired: 1 in]
            n156 = shared-variable ".\\Shared Variables.lvlib\\Elevator.lvlib\\Elevator Response"(error in=w334) -> (w327:dbl)  [unwired: 1 out]
            n157 = Replace Array Subset(array=w330, new element #1=w329, index #1=0 ("index"), new element #2=w328, index #2=1 ("index"), new element #3=w327, index #3=2 ("index")) -> (w325:dbl[])
            n158 = Enqueue Element(queue=w326, element=w325) -> ()  [unwired: 2 in, 3 out]
          }
        }
        n159 = case shown="True" w302 {
          tunnel: w306 -> [_ w319]
          tunnel: w304 -> [_ w317]
          tunnel: w301 -> [_ w316]
          frame False {
            # "Logging to TDMS is Off while collecting data for next Burst"
          }
          frame True {
            # "Burst data to TDMS"
            n160 = for {
              N: w316 -> [_]
              tunnel: [w324] -> w318 mode=indexing
              tunnel: w317 -> [w323]
              n161 = Dequeue Element(queue=w323) -> (element=w324:dbl[])  [unwired: 2 in, 3 out]
            }
            n162 = TDMS Write(0:w319, 1:enum16{"decimated", "interleaved"}."interleaved" ("data layout (0:decimated)"), 5:"Shooter" ("group name in (Untitled)"), 7:string[] ["Time", "RPM", "Elevator"] ("channel name(s) in (Untitled)"), 9:w318) -> ()  [unwired: 1 in, 4 out]
          }
        }
      }
    }
    n163 = Wait (ms)(milliseconds to wait=u32 51) -> ()  [unwired: 1 out]
  }
  n164 = while "Current Sensor Logging Loop" {
    tunnel: w43 -> [w339]
    tunnel: w39 -> [w343]
    tunnel: w38 -> [w342]
    tunnel: w35 -> [w341]
    tunnel: w34 -> [w336]
    stop <- FALSE stop-if-true
    n165 = shared-variable ".\\Shared Variables.lvlib\\System.lvlib\\Data Log"() -> (w338:bool)  [unwired: 1 in, 1 out]
    n166 = And(x="Log Enable", y=w338) -> (x .and. y?=w340:bool)
    n167 = case shown="True" w340 {
      tunnel: w339 -> [_ w356]
      tunnel: w343 -> [_ w353]
      tunnel: w342 -> [_ w352]
      tunnel: w341 -> [_ w349]
      tunnel: w336 -> [_ w347]
      frame False {
        # "Logging is disabled"
      }
      frame True {
        w345 = 90 ("y")
        n168 = Get Date/Time In Seconds() -> (seconds since 1Jan1904=w360:timestamp)
        n169 = Get Queue Status(queue=w352) -> (queue out=w351:refnum<queue>, # elements in queue=w346:i32)  [unwired: 2 in, 6 out]
        "# elements in queue 2" <- w346
        "Q 2" <- w346
        n170 = To Double Precision Float(number=w360) -> (double precision float=w359:dbl)
        n171 = Greater Or Equal?(x=w346, y=w345) -> (x >= y?=w350:bool)
        n172 = Subtract(x=w359, y=w356) -> (x-y=w355:dbl)
        n173 = Quotient & Remainder(x=w355, y="Sample (s)") -> (floor(x/y)=w357:dbl)  [unwired: 1 out]
        n174 = feedback #6() -> (w358:dbl)  [unwired: 1 in]
        n175 = feedback-in #6(w357) -> ()
        n176 = Greater?(x=w357, y=w358) -> (0:w354:bool)
        n177 = case shown="True" w354 {
          tunnel: w355 -> [_ w374]
          tunnel: w353 -> [_ w376]
          tunnel: w352 -> [_ w386]
          tunnel: w349 -> [_ w373]
          frame False {
            # "Logging to Queue is Off during not-sample time period"
          }
          frame True {
            # "Queue up data at Sample time"
            n178 = call <vilib>:"WPI_AnalogChannelGetAverageVoltage.vi"("AIDeviceRef"=w373) -> ("Voltage"=w370:dbl)  [unwired: 8 in, 2 out]
            n179 = shared-variable ".\\Shared Variables.lvlib\\Ascent.lvlib\\Climb Mode"() -> (w377:u16, error out=w385:errorcluster)  [unwired: 1 in]
            n180 = shared-variable ".\\Shared Variables.lvlib\\Ascent.lvlib\\Climb Step"(error in=w385) -> (w378:i32)  [unwired: 1 out]
            n181 = Multiply(x="A / V", y=w370) -> (x*y=→"Current":dbl)
            n182 = To Double Precision Float(number=w377) -> (double precision float=w383:dbl)
            n183 = To Double Precision Float(number=w378) -> (double precision float=w384:dbl)
            n184 = Replace Array Subset(array=w376, new element #1=w374, index #1=0 ("index"), new element #2=w370, index #2=1 ("index"), new element #3=w383, index #3=2 ("index"), new element #4=w384, index #4=3 ("index")) -> (w375:dbl[])
            n185 = Enqueue Element(queue=w386, element=w375) -> ()  [unwired: 2 in, 3 out]
          }
        }
        n186 = case shown="True" w350 {
          tunnel: w351 -> [_ w364]
          tunnel: w345 -> [_ w363]
          tunnel: w347 -> [_ w361]
          frame False {
            # "Logging to TDMS is Off while collecting data for next Burst"
          }
          frame True {
            # "Burst data to TDMS"
            n187 = for {
              N: w363 -> [_]
              tunnel: [w369] -> w365 mode=indexing
              tunnel: w364 -> [w368]
              n188 = Dequeue Element(queue=w368) -> (element=w369:dbl[])  [unwired: 2 in, 3 out]
            }
            n189 = TDMS Write(0:w361, 1:enum16{"decimated", "interleaved"}."interleaved" ("data layout (0:decimated)"), 5:"Current" ("group name in (Untitled)"), 7:string[] ["Time", "Avg Volts", "Mode", "Step", ""] ("channel name(s) in (Untitled)"), 9:w365) -> ()  [unwired: 1 in, 4 out]
          }
        }
      }
    }
    n190 = Wait (ms)(milliseconds to wait=u32 9) -> ()  [unwired: 1 out]
  }
  n191 = while "Fire Control Logging Loop" {
    tunnel: w116 -> [w395]
    tunnel: w112 -> [w394]
    tunnel: w34 -> [w393]
    i -> [w392]
    stop <- FALSE stop-if-true
    n192 = call "Elapsed Times.vi"("Call Name"="Log") -> ()  [unwired: 2 in, 1 out]
    n193 = local read "Save"() -> (w390:bool)
    n194 = call "Fire Data Logger.vi"("Save"=w390, "Init Array"=w394, "Burst"="Burst", "rt fifo"=w395, "TDMS Refnum"=w393) -> ()  [unwired: 7 in]
    n195 = Wait (ms)(milliseconds to wait="loop period (ms)") -> ()  [unwired: 1 out]
    "iterations" <- w392
  }
  n196 = call <vilib>:"WPI_RelayRefNum Registry Get.vi"("refnum name"="compressor") -> ("RelayDevRef"=w120:T24)  [unwired: 9 in, 1 out]
  n197 = while "Compressor Control Loop" {
    tunnel: w120 -> [w404]
    tunnel: w132 -> [w402]
    stop <- FALSE stop-if-true
    n198 = call <vilib>:"WPI_DigitalInputGetValue.vi"("DigitalInputDevRef"=w402) -> ("Value"=w397:bool)  [unwired: 8 in, 2 out]
    n199 = Not(x=w397) -> (.not. x?=w400:bool)
    "Compressor Running" <- w400
    n200 = Select(t=WPI_RelayValue."Off" ("RelayValue"), s=w397, f=WPI_RelayValue."Forward" ("RelayValue")) -> (s? t:f=w396:T37)
    n201 = Build Array(w400) -> (w401:bool[])
    n202 = call <vilib>:"WPI_RelaySet.vi"("RelayValue"=w396, "RelayDevRef"=w404) -> ()  [unwired: 8 in, 2 out]
    n203 = call <vilib>:"WPI_DriverStationSet Digital Output.vi"("Driver Station Digital Output (1-8)"=w401) -> ()  [unwired: 10 in, 1 out]
    n204 = Wait (ms)(milliseconds to wait=u32 300) -> ()  [unwired: 1 out]
  }
  n205 = call <vilib>:"WPI_ServoRefNum Registry Get.vi"("refnum name"="brakeServo") -> ("ServoDeviceRef"=w21:T38)  [unwired: 9 in, 1 out]
  n206 = call <vilib>:"WPI_EncoderRefNum Registry Get.vi"("refnum name"="climbSensor") -> ("EncoderDevRef"=w28:T18)  [unwired: 9 in, 1 out]
  n207 = call <vilib>:"WPI_MotorControlRefNum Registry Get.vi"("refnum name"="climbMotor") -> ("MotorControlDevRef"=w15:T8)  [unwired: 9 in, 1 out]
  n208 = call <vilib>:"WPI_DigitalInputRefNum Registry Get.vi"("refnum name"="skyHookHome") -> ("DigitalInputDevRef"=w11:T27)  [unwired: 9 in, 1 out]
  n209 = call <vilib>:"WPI_SolenoidRefNum Registry Get.vi"("refnum name"="slapper") -> ("SolenoidDevRef"=w17:T21)  [unwired: 9 in, 1 out]
  n210 = call <vilib>:"WPI_AnalogChannelRefNum Registry Get.vi"("refnum name"="climbMotorCurrent") -> ("AIDeviceRef"=w25:T32)  [unwired: 9 in, 1 out]
  n211 = call <vilib>:"WPI_SolenoidRefNum Registry Get.vi"("refnum name"="pullUp") -> ("SolenoidDevRef"=w23:T21)  [unwired: 9 in, 1 out]
  n212 = node-c288(w88) -> ()  [unwired: 1 out]
  n213 = Get Date/Time In Seconds() -> (seconds since 1Jan1904=w69:timestamp)
  n214 = Get Date/Time In Seconds() -> (seconds since 1Jan1904=w4:timestamp)
  n215 = To Double Precision Float(number=w69) -> (double precision float=w68:dbl)
  n216 = while "Wheel Encoder Read Loop" {
    tunnel: w74 -> [w434]
    tunnel: w73 -> [w433]
    tunnel: w33 -> [w423]
    tunnel: w68 -> [w424]
    tunnel: w70 -> [w415]
    stop <- FALSE stop-if-true
    n217 = call <vilib>:"WPI_EncoderGet.vi"("EncoderDevRef"=w433) -> ("Distance"=w411:dbl, "Stopped"=→"RStopped":bool)  [unwired: 5 in, 4 out]
    "Right Wheel Encoder" <- w411
    n218 = call <vilib>:"WPI_EncoderGet.vi"("EncoderDevRef"=w434) -> ("Distance"=w412:dbl, "Stopped"=→"LStopped":bool)  [unwired: 5 in, 4 out]
    "Left Wheel Encoder" <- w412
    n219 = disable-structure shown="Disabled" {
      disable-tunnel: w415 -> [w442 _]
      frame Disabled {
        n220 = call <vilib>:"WPI_GyroSetGain.vi"("Gain (VoltsPerDegree/Second)"="Gyro Gain (VoltsPerDegree/Second)", "GyroDevRef"=w442) -> ("error out"=w441:errorcluster, "GyroDevRef"=w440:T15)  [unwired: 8 in]
        n221 = call <vilib>:"WPI_GyroGetAngle.vi"("error in (no error)"=w441, "GyroDevRef"=w440) -> ("Angle"=→"Angle":dbl)  [unwired: 6 in, 3 out]
      }
      frame Enabled {
      }
    }
    n222 = Add(x=w412, y=w411) -> (x+y=w436:dbl)
    n223 = shared-variable ".\\Shared Variables.lvlib\\Sensors.lvlib\\LeftWheelEncoder"(w412) -> (error out=w407:errorcluster)  [unwired: 1 in]
    n224 = Divide(x=w436, y=2.0) -> (x/y=w410:dbl)
    n225 = shared-variable ".\\Shared Variables.lvlib\\Sensors.lvlib\\AvgWheelEncoder"(w410, error in=w407) -> (error out=w406:errorcluster)
    n226 = shared-variable ".\\Shared Variables.lvlib\\Sensors.lvlib\\RightWheel Encoder"(w411, error in=w406) -> ()  [unwired: 1 out]
    n227 = feedback #7() -> (w421:dbl)  [unwired: 1 in]
    n228 = feedback-in #7(w411) -> ()
    n229 = Not Equal?(x=w411, y=w421) -> (x != y?=w419:bool)
    n230 = Get Date/Time In Seconds() -> (seconds since 1Jan1904=w429:timestamp)
    n231 = feedback-in #8(w412) -> ()
    n232 = feedback #8() -> (w422:dbl)  [unwired: 1 in]
    n233 = To Double Precision Float(number=w429) -> (double precision float=w428:dbl)
    n234 = Not Equal?(x=w412, y=w422) -> (x != y?=w420:bool)
    n235 = Subtract(x=w428, y=w424) -> (x-y=w427:dbl)
    n236 = Quotient & Remainder(x=w427, y="Sample Rate (sec)") -> (floor(x/y)=w425:dbl)  [unwired: 1 out]
    n237 = feedback #9() -> (w426:dbl)  [unwired: 1 in]
    n238 = feedback-in #9(w425) -> ()
    n239 = Or(x=w420, y=w419) -> (x .or. y?=w418:bool)
    n240 = Greater?(x=w425, y=w426) -> (0:w417:bool)
    n241 = And(x=w418, y=w417) -> (x .and. y?=w416:bool)
    n242 = Select(t=w416, s="Sample?", f=TRUE) -> (s? t:f=w409:bool)
    n243 = case shown="True" w409 {
      tunnel: w412 -> [_ w452]
      tunnel: w411 -> [_ w450]
      tunnel: w429 -> [_ w459]
      tunnel: w423 -> [_ w448]
      frame False {
        # "Odometer Logging is Off"
      }
      frame True {
        n244 = shared-variable ".\\Shared Variables.lvlib\\Sensors.lvlib\\Left Odo"() -> (w445:dbl, error out=w443:errorcluster)  [unwired: 1 in]
        "Left Odometer" <- w445
        n245 = shared-variable ".\\Shared Variables.lvlib\\Sensors.lvlib\\Right Odo"(error in=w443) -> (w444:dbl)  [unwired: 1 out]
        "Right Odometer" <- w444
        n246 = Add(x=w450, y=w444) -> (x+y=w449:dbl)
        n247 = Add(x=w445, y=w452) -> (x+y=w451:dbl)
        n248 = Build Array(w451, w449) -> (w456:dbl[])
        n249 = Build Array(w459) -> (w460:timestamp[])
        n250 = TDMS Write(0:w448, 1:enum16{"decimated", "interleaved"}."interleaved" ("data layout (0:decimated)"), 5:"Odometer" ("group name in (Untitled)"), 7:string[] ["Time"] ("channel name(s) in (Untitled)"), 9:w460) -> (4:w458:refnum<k34>, 6:w457:string)  [unwired: 1 in, 2 out]
        n251 = TDMS Write(0:w458, 1:enum16{"decimated", "interleaved"}."interleaved" ("data layout (0:decimated)"), 5:w457, 7:string[] ["Left Enc", "Right Enc"] ("channel name(s) in (Untitled)"), 9:w456) -> ()  [unwired: 1 in, 4 out]
      }
    }
    n252 = Wait (ms)(milliseconds to wait="enc ms to wait") -> ()  [unwired: 1 out]
  }
  n253 = To Double Precision Float(number=w4) -> (double precision float=w3:dbl)
  n254 = timed-loop "Auto Ascent Loop\nTime Critical" {
    tunnel: w17 -> [w468]
    tunnel: w15 -> [w480]
    tunnel: w23 -> [w476]
    tunnel: w28 -> [w481]
    tunnel: w25 -> [w482]
    shift-right: [w483] -> _
    shift-left: w13 -> [w467]
    shift-left: w13 -> [w466]
    tunnel: w11 -> [w479]
    timing: w30 -> [_]
    timing-out: [_] -> w29
    tunnel: w21 -> [w472]
    tunnel: w18 -> [w475]
    tunnel: w19 -> [w469]
    tunnel: w3 -> [w470]
    shift-right: [w465] -> _
    shift-left: 0.0 ("Time Out") -> [w464]
    shift-right: [w463] -> _
    shift-left: 0 ("Rung counter out") -> [w462]
    stop <- FALSE stop-if-true
    n255 = shared-variable ".\\Shared Variables.lvlib\\Ascent.lvlib\\Climb Step"(w467) -> ()  [unwired: 1 in, 1 out]
    n256 = call "Elapsed Times.vi"("Call Name"="Climb") -> ()  [unwired: 2 in, 1 out]
    n257 = local read "Burst"() -> (w474:i32)
    n258 = shared-variable ".\\Shared Variables.lvlib\\Ascent.lvlib\\Climb Mode"() -> (w478:u16)  [unwired: 1 in, 1 out]
    n259 = call "Climb Loop.vi"("ClimbMotor"=w480, "SkyHome"=w479, "Slapper"=w468, "Climb Step In"=w467, "Climb Step In2"=w466, "Time In"=w464, "ClimbEncoder"=w481, "Rung counter in"=w462, "BrakeServo"=w472, "PullUp"=w476, "array"=w475, "ClimbCurrent"=w482, "rt fifo"=w469, "Auto Ascent Log Enable"="Auto Ascent Log Enable", "time ref"=w470, "Climb mode In"=w478) -> ("Rung counter out"=w463:i32, "Climb Step Out"=w483:T1, "# elements"=w461:u32, "Time Out"=w465:dbl)
    "FIFO Elements" <- w461
    n260 = Greater?(x=w461, y=w474) -> (0:→"Save Ascent":bool)
  }
  n261 = node-c288(w29) -> ()  [unwired: 1 out]
  n262 = node-c288(i64 21 ("Period")) -> (w64:T29)  [unwired: 3 in]
  n263 = call <vilib>:"WPI_AnalogChannelRefNum Registry Get.vi"("refnum name"="Sonar") -> ("AIDeviceRef"=w77:T32)  [unwired: 1 in, 9 out]
  n264 = call <vilib>:"WPI_RobotDriveRefNum Registry Get.vi"("refnum name"="robotDrive") -> ("RobotDriveDevRef"=w79:T39)  [unwired: 9 in, 1 out]
  n265 = call <vilib>:"WPI_AnalogChannelRefNum Registry Get.vi"("refnum name"="elevatorEncoder") -> ("AIDeviceRef"=w59:T32)  [unwired: 9 in, 1 out]
  n266 = node-c288(i64 41 ("Period")) -> (w82:T29)  [unwired: 3 in]
  n267 = while "Ascent, Supervisory Control Loop" {
    shift-right: [w488] -> _
    shift-left: enum16{"Wait", "Automatic", "Manual", "Abort"}."Wait" ("Climb mode") -> [w487]
    stop <- FALSE stop-if-true
    # "States\n0:  Wait\n1:  Automatic\n2:  Manual\n3:  Abort"
    # "Button 9 controls the mode \nFirst press ---- Starts the climb (deploys mechinism)\nSecond press --- Exits auto climb and allows for manual control\nThird press ---- Abort mode there is no possible action from here"
    n268 = shared-variable ".\\Shared Variables.lvlib\\Gamepad Driver.lvlib\\Dr Button 9"() -> (w490:bool)  [unwired: 1 in, 1 out]
    n269 = shared-variable ".\\Shared Variables.lvlib\\Gamepad Driver.lvlib\\Dr Button 10"() -> (w489:bool)  [unwired: 1 in, 1 out]
    n270 = feedback #10(FALSE ("Button 1")) -> (w495:bool)
    n271 = feedback-in #10(w490) -> ()
    n272 = Greater?(x=w490, y=w495) -> (0:w491:bool)
    n273 = case shown="\"Wait\"" w487 {
      selector: w487 -> [w502 w508 w515 w521]
      tunnel: [w497 w507 w514 w524] -> w488
      tunnel: w491 -> [w501 _ _ w523]
      tunnel: w489 -> [w496 w506 _ _]
      frame "Automatic", Default {
        # "This is the abort button, it should perform a \nmaster abort no matter what climb mode or\nclimb step we are in."
        n274 = Select(t=enum16{"Wait", "Automatic", "Manual", "Abort"}."Manual" ("Climb mode"), s=w501, f=w502) -> (s? t:f=w500:enum16{"Wait", "Automatic", "Manual", "Abort"})
        n275 = feedback #11(FALSE ("Button 1")) -> (w504:bool)
        n276 = feedback-in #11(w496) -> ()
        n277 = Greater?(x=w496, y=w504) -> (0:w498:bool)
        n278 = Select(t=enum16{"Wait", "Automatic", "Manual", "Abort"}."Abort" ("Climb mode"), s=w498, f=w500) -> (s? t:f=w497:enum16{"Wait", "Automatic", "Manual", "Abort"})
      }
      frame "Manual" {
        n279 = feedback #12(FALSE ("Button 1")) -> (w511:bool)
        n280 = feedback-in #12(w506) -> ()
        n281 = Greater?(x=w506, y=w511) -> (0:w509:bool)
        n282 = Select(t=enum16{"Wait", "Automatic", "Manual", "Abort"}."Automatic" ("Climb mode"), s=w509, f=w508) -> (s? t:f=w507:enum16{"Wait", "Automatic", "Manual", "Abort"})
      }
      frame "Abort" {
        n283 = shared-variable ".\\Shared Variables.lvlib\\Gamepad Driver.lvlib\\Dr Button 10"() -> (w513:bool)  [unwired: 1 in, 1 out]
        n284 = feedback #13(FALSE ("Button 1")) -> (w518:bool)
        n285 = feedback-in #13(w513) -> ()
        n286 = Greater?(x=w513, y=w518) -> (0:w516:bool)
        n287 = Select(t=enum16{"Wait", "Automatic", "Manual", "Abort"}."Manual" ("Climb mode"), s=w516, f=w515) -> (s? t:f=w514:enum16{"Wait", "Automatic", "Manual", "Abort"})
      }
      frame "Wait" {
        # "This is the starting case that keeps \nall buttons except for button 9\ninactive untill a climb has started"
        n288 = shared-variable ".\\Shared Variables.lvlib\\Ascent.lvlib\\Climb Started"(FALSE ("Climb Started x")) -> ()  [unwired: 1 in, 1 out]
        n289 = Select(t=enum16{"Wait", "Automatic", "Manual", "Abort"}."Automatic" ("Climb mode"), s=w523, f=w521) -> (s? t:f=w524:enum16{"Wait", "Automatic", "Manual", "Abort"})
      }
    }
    n290 = shared-variable ".\\Shared Variables.lvlib\\Ascent.lvlib\\Climb Mode"(w488) -> ()  [unwired: 1 in, 1 out]
    n291 = Wait (ms)(milliseconds to wait=u32 100) -> ()  [unwired: 1 out]
  }
  n292 = node-c288(w109) -> ()  [unwired: 1 out]
  n293 = timed-loop "Drive Motor Loop\nTime Critical" {
    tunnel: w79 -> [w525]
    tunnel: w77 -> [w526]
    timing: w82 -> [_]
    timing-out: [_] -> w81
    stop <- FALSE stop-if-true
    n294 = call "Elapsed Times.vi"("Call Name"="Drive") -> ()  [unwired: 2 in, 1 out]
    n295 = call "Drive Loop.vi"("RobotDriveDevRef"=w525, "Sonar"=w526) -> ()  [unwired: 1 in]
  }
  n296 = call <vilib>:"WPI_MotorControlRefNum Registry Get.vi"("refnum name"="shooterElevator") -> ("MotorControlDevRef"=w58:T8)  [unwired: 9 in, 1 out]
  n297 = timed-loop "Elevator Control Loop\nTime Critical" {
    tunnel: w58 -> [w532]
    tunnel: w59 -> [w533]
    tunnel: "Elev Stable Tol (sec)" -> [w531]
    tunnel: w119 -> [w534]
    timing: w64 -> [_]
    timing-out: [_] -> w63
    stop <- FALSE stop-if-true
    n298 = call "Elevator Loop.vi"("Elevator Enc"=w533, "Elevator"=w532, "Personality"=w534, "Elev Stable Tol (sec)"=w531, "Auto Pitch"="Auto Pitch") -> ()  [unwired: 1 in]
    n299 = call "Elapsed Times.vi"("Call Name"="El") -> ()  [unwired: 2 in, 1 out]
  }
  n300 = node-c288(w81) -> ()  [unwired: 1 out]
  n301 = node-c288(w63) -> ()  [unwired: 1 out]
  n302 = while "Log Key Parameters" {
    tunnel: w34 -> [w544]
    tunnel: w95 -> [_]
    stop <- TRUE stop-if-true
    # "Channel ID"
    # "Group ID"
    n303 = shared-variable ".\\Shared Variables.lvlib\\Shooter.lvlib\\Shooter Tolerance"() -> (w541:dbl)  [unwired: 1 in, 1 out]
    n304 = shared-variable ".\\Shared Variables.lvlib\\Elevator.lvlib\\Std Pitch"() -> (w542:dbl)  [unwired: 1 in, 1 out]
    n305 = shared-variable ".\\Shared Variables.lvlib\\Shooter.lvlib\\Std RPM"() -> (w543:dbl)  [unwired: 1 in, 1 out]
    n306 = Build Array(w543, w542, w541) -> (w547:dbl[])
    n307 = TDMS Write(0:w544, 1:enum16{"decimated", "interleaved"}."interleaved" ("data layout (0:decimated)"), 5:"Parameters" ("group name in (Untitled)"), 7:string[] ["Tele RPM", "Tele Pitch", "Tele RPM Tolerance", ""] ("channel name(s) in (Untitled)"), 9:w547) -> ()  [unwired: 1 in, 4 out]
  }
  n308 = disable-structure shown="Disabled" {
    disable-tunnel: [w551 _] -> w32
    disable-tunnel: [w550 _] -> w31
    frame Disabled {
      n309 = Initialize Array(0.0 ("element"), 9 ("dimension size")) -> (w550:dbl[])
      n310 = Obtain Queue(name (unnamed)="Q", element data type=w550) -> (queue out=w551:refnum<queue>)  [unwired: 3 in, 2 out]
      n311 = TDMS Open(7:enum16{"1.0", "2.0"}."2.0" ("file format version (2.0)"), 10:T4."open or create" ("operation (0:open)"), 11:path "C:/tmp/Ascent B.tdms" ("file path (dialog if empty)")) -> (3:w559:refnum<k34>)  [unwired: 3 in, 1 out]
      n312 = while {
        tunnel: w559 -> [w563]
        tunnel: w551 -> [w570]
        tunnel: [w568] -> w556
        tunnel: [w563] -> w555
        stop <- FALSE stop-if-true
        w565 = 50 ("y")
        n313 = Get Queue Status(queue=w570) -> (queue out=w568:refnum<queue>, # elements in queue=w567:i32)  [unwired: 2 in, 6 out]
        "# elements in queue 3" <- w567
        n314 = Greater Or Equal?(x=w567, y=w565) -> (x >= y?=w566:bool)
        n315 = case shown="True" w566 {
          tunnel: w568 -> [_ w577]
          tunnel: w565 -> [_ w576]
          tunnel: w563 -> [_ w573]
          tunnel: string[] ["Iteration", "Position", "Gear", "Rate", "Rate offset", "Set", "Reset", "Q", "Motor"] ("channel name(s) in (Untitled)") -> [_ w572]
          frame False {
          }
          frame True {
            n316 = for {
              N: w576 -> [_]
              tunnel: [w579] -> w574 mode=indexing
              tunnel: w577 -> [w578]
              n317 = Dequeue Element(queue=w578) -> (element=w579:dbl[])  [unwired: 2 in, 3 out]
            }
            n318 = TDMS Write(0:w573, 1:enum16{"decimated", "interleaved"}."interleaved" ("data layout (0:decimated)"), 5:"Group" ("group name in (Untitled)"), 7:w572, 9:w574) -> ()  [unwired: 1 in, 4 out]
          }
        }
        n319 = Wait (ms)(milliseconds to wait=u32 20) -> ()  [unwired: 1 out]
      }
      n320 = Flush Queue(queue=w556) -> (queue out=w558:refnum<queue>, error out=w557:errorcluster)  [unwired: 1 in, 1 out]
      n321 = TDMS Close(11:w555) -> ()  [unwired: 1 in, 2 out]
      n322 = Release Queue(queue=w558, error in (no error)=w557) -> ()  [unwired: 1 in, 3 out]
    }
    frame Enabled {
    }
  }
  n323 = disable-structure shown="Disabled" {
    disable-tunnel: w32 -> [w581 _]
    disable-tunnel: w31 -> [w580 _]
    frame Disabled {
      # "Brake"
      n324 = node-c288() -> (w592:T29)  [unwired: 4 in]
      n325 = call <vilib>:"WPI_DigitalInputRefNum Registry Get.vi"("refnum name"="skyHookHome") -> ("DigitalInputDevRef"=w582:T27)  [unwired: 9 in, 1 out]
      n326 = call <vilib>:"WPI_EncoderRefNum Registry Get.vi"("refnum name"="climbSensor") -> ("EncoderDevRef"=w583:T18)  [unwired: 9 in, 1 out]
      n327 = call <vilib>:"WPI_MotorControlRefNum Registry Get.vi"("refnum name"="climbMotor") -> ("MotorControlDevRef"=w584:T8)  [unwired: 9 in, 1 out]
      n328 = timed-loop {
        tunnel: w584 -> [w616]
        tunnel: w583 -> [w615]
        tunnel: w582 -> [w614]
        timing: w592 -> [_]
        timing-out: [_] -> w591
        tunnel: w581 -> [w595]
        tunnel: w580 -> [w594]
        i -> [w596]
        stop <- FALSE stop-if-true
        n329 = call <vilib>:"WPI_DigitalInputGetValue.vi"("DigitalInputDevRef"=w614) -> ("Value"=w613:bool)  [unwired: 8 in, 2 out]
        n330 = call <vilib>:"WPI_EncoderGet.vi"("EncoderDevRef"=w615) -> ("Distance"=w601:dbl, "Rate"=w602:dbl)  [unwired: 5 in, 4 out]
        "Distance" <- w601
        "Rate" <- w602
        n331 = Not(x=w613) -> (.not. x?=→"Home":bool)
        n332 = case shown="False" "PID" {
          tunnel: [w631 w633] -> _
          tunnel: w601 -> [w630 w639]
          tunnel: "SkyHook" -> [w621 _]
          tunnel: "Motor Coerce" -> [w618 w634]
          frame False {
            n333 = Greater Than 0?(x=w621) -> (x > 0?=w620:bool)
            n334 = Select(t="Speed near Lim Up", s=w620, f="Speed near Lim Dn") -> (s? t:f=w622:dbl)
            n335 = call "Soft Stops.vi"("Motor In"=w621, "correlation"=TRUE, "Sense"=w630, "Lo Limit"="Lo Limit", "Hi Limit"="Hi Limit", "Speed near Limit"=w622, "Margin"="Near Limit", "Motor Coerce"=w618) -> ("Motor Out"=w631:dbl, "At Lo"=→"At Lo":bool, "At Hi"=→"At Hi":bool)  [unwired: 5 in]
          }
          frame True {
            n336 = Subtract(x="Position", y=w639) -> (x-y=w638:dbl)
            "err" <- w638
            n337 = Multiply(x=w638, y="P") -> (x*y=w636:dbl)
            n338 = Negate(x=w634) -> (-x=w635:dbl)
            n339 = In Range and Coerce(upper limit=w634, x=w636, lower limit=w635) -> (coerced(x)=w633:dbl)  [unwired: 1 out]
          }
        }
        n340 = Bundle("Rate"=w602, "Distance"=w601) -> (→"Rate":cluster{"Rate":dbl, "Distance":dbl})  [unwired: 1 in]
        n341 = call "Velocity Profile.vi"("Set Point"="Set Point", "Iteration"=w596, "Reset"="Reset", "Reset 2"="Reset 2", "Position Sense"=w601, "Rate Sense"=w602, "Velocity Profile"="Velocity Profile", "queue"=w595, "Hold"="Hold", "array"=w594) -> ("Motor"=w599:dbl, "arrived"=→"arrived":bool, "gear"=w604:i32)  [unwired: 3 in]
        "Motor" <- w599
        "val" <- w599
        "gear" <- w604
        n342 = call "SimpleSetMotor.vi"("Output"=w599, "MotorControlDevRef"=w616) -> ()  [unwired: 8 in, 2 out]
        n343 = disable-structure shown="Disabled" {
          frame Disabled {
            n344 = Wait (ms)(milliseconds to wait=u32 51) -> ()  [unwired: 1 out]
          }
          frame Enabled {
          }
        }
        n345 = Bundle("Motor"=w599, "gear"=w604) -> (→"motor":cluster{"Motor":dbl, "gear":i32})  [unwired: 1 in]
        n346 = node-c288("Period") -> ()  [unwired: 1 in, 1 out]
      }
      n347 = call <vilib>:"WPI_ServoRefNum Registry Get.vi"("refnum name"="brakeServo") -> ("ServoDeviceRef"=w588:T38)  [unwired: 9 in, 1 out]
      n348 = call <vilib>:"WPI_ServoSetAngle.vi"("Angle"=0, "ServoDeviceRef"=w588) -> ()  [unwired: 8 in, 2 out]
      n349 = node-c288(w591) -> ()  [unwired: 1 out]
    }
    frame Enabled {
    }
  }
  n350 = disable-structure shown="Disabled" {
    frame Disabled {
      w657 = climb_step_state."Approach Bar" ("Climb Step")
      # "Auto Ascent Loop"
      # "When the button is pressed the first time the climb starts,\nif the button is pressed again the climb is aborted."
      n351 = call <vilib>:"WPI_DigitalInputRefNum Registry Get.vi"("refnum name"="skyHookHome") -> ("DigitalInputDevRef"=w659:T27)  [unwired: 9 in, 1 out]
      n352 = call <vilib>:"WPI_AnalogChannelRefNum Registry Get.vi"("refnum name"="climbMotorCurrent") -> ("AIDeviceRef"=w654:T32)  [unwired: 9 in, 1 out]
      n353 = call <vilib>:"WPI_EncoderRefNum Registry Get.vi"("refnum name"="climbSensor") -> ("EncoderDevRef"=w651:T18)  [unwired: 9 in, 1 out]
      n354 = call <vilib>:"WPI_SolenoidRefNum Registry Get.vi"("refnum name"="pullUp") -> ("SolenoidDevRef"=w656:T21)  [unwired: 9 in, 1 out]
      n355 = call <vilib>:"WPI_MotorControlRefNum Registry Get.vi"("refnum name"="climbMotor") -> ("MotorControlDevRef"=w649:T8)  [unwired: 9 in, 1 out]
      n356 = call <vilib>:"WPI_SolenoidRefNum Registry Get.vi"("refnum name"="slapper") -> ("SolenoidDevRef"=w647:T21)  [unwired: 9 in, 1 out]
      n357 = while {
        tunnel: w647 -> [w686]
        tunnel: w649 -> [w687]
        tunnel: w656 -> [w688]
        tunnel: w651 -> [w660]
        tunnel: w654 -> [w685]
        shift-right: [w683] -> _
        shift-left: w657 -> [w681]
        shift-left: w657 -> [w682]
        tunnel: w659 -> [w675]
        stop <- FALSE stop-if-true
        n358 = shared-variable ".\\Shared Variables.lvlib\\Ascent.lvlib\\Climb Mode"() -> (w661:u16)  [unwired: 1 in, 1 out]
        "Climb mode 2" <- w661
        n359 = case shown="3" w661 {
          tunnel: ["Wait" "Automatic" "Manual" "Abort"] -> w679
          frame 0, Default {
          }
          frame 1 {
          }
          frame 2 {
          }
          frame 3 {
          }
        }
        n360 = call <vilib>:"WPI_DigitalInputGetValue.vi"("DigitalInputDevRef"=w675) -> ("Value"=w673:bool)  [unwired: 8 in, 2 out]
        n361 = feedback-in #14(w673) -> ()
        n362 = feedback #14() -> (w674:bool)  [unwired: 1 in]
        n363 = call <vilib>:"SD Write String.vi"("String"=w679, "Name"="climbMode_i") -> ()  [unwired: 8 in, 2 out]
        n364 = Greater?(x=w673, y=w674) -> (0:w672:bool)
        n365 = Less?(x=w673, y=w674) -> (x < y?=w671:bool)
        n366 = Or(x=w672, y=w671) -> (x .or. y?=w666:bool)
        n367 = call <vilib>:"WPI_EncoderGet.vi"("EncoderDevRef"=w660) -> ("Distance"=w667:dbl)  [unwired: 5 in, 5 out]
        "Sky Enc 2" <- w667
        n368 = case shown="1" w661 {
          tunnel: w688 -> [w708 _ _ w852]
          tunnel: w687 -> [w707 _ w840 w851]
          tunnel: w660 -> [w706 _ w841 _]
          tunnel: w686 -> [w705 _ _ w853]
          tunnel: w685 -> [w704 _ _ _]
          tunnel: [w703 climb_step_state."Abort" ("Climb Step") climb_step_state."Approach Bar" ("Climb Step") climb_step_state."Abort" ("Climb Step")] -> w683
          tunnel: w681 -> [w702 _ _ _]
          tunnel: w682 -> [w701 _ _ _]
          tunnel: "Climb Extend Tail Speed 2" -> [w700 _ _ w849]
          tunnel: "Climb Retract Tail Speed 2" -> [w699 _ _ w848]
          tunnel: "Man Flip Speed 2" -> [w698 _ _ w847]
          tunnel: "Slow Extend 2" -> [_ _ _ w846]
          tunnel: "Slow Retract 2" -> [_ _ _ w845]
          frame 1 {
            # "2/11/12 -- ZL: Replaced Local enum with a \ntypedef to add a state change the \ntypedef called: Climb Step Control"
            # "When the button to start the climb is pressed the\nfirst time the outside case statement becomes true,\nthen the inside case statement is true for the first\niteration of the while loop. After the first iteration\nthe inside case statement turns false and takes the\nvalue of from the shift register (determined by the\nlarge case statement) and is used to control the \nlarge case statement. If the button is pressed again \nthen the large case statement turns to false and \nswitches the large case statement to the abort\ncase."
            n369 = case shown="\"Approach +\"" w702 {
              selector: w702 -> [_ _ _ _ w748 _ w760 _ w784 _ w811]
              tunnel: w708 -> [w711 w730 _ w744 _ _ _ w770 w788 _ _]
              tunnel: [climb_step_state."Abort" ("Climb Step") w718 w731 climb_step_state."Check Continue" ("Climb Step") w750 climb_step_state."Climb Step 4" ("Climb Step") w762 w769 w785 w800 w812] -> w703
              tunnel: w707 -> [w715 w727 w734 _ w751 _ w765 _ w790 _ _]
              tunnel: w706 -> [_ w726 w733 _ _ _ _ _ w794 _ _]
              tunnel: w705 -> [w713 _ _ _ _ w757 _ w771 _ _ _]
              tunnel: w704 -> [_ _ _ _ _ _ _ w775 _ _ _]
              tunnel: w701 -> [_ _ _ _ _ _ _ _ _ _ w807]
              tunnel: w700 -> [_ _ w732 _ w747 _ _ _ _ _ _]
              tunnel: w699 -> [_ _ _ _ _ _ _ _ w783 _ _]
              tunnel: w698 -> [_ _ _ _ _ _ _ _ _ _ _]
              frame "Abort" {
                # "In this case all outputs should be set to 0 or un engaged"
                n370 = call <vilib>:"WPI_MotorControlSetOutput.vi"("Output"=0.0, "MotorControlDevRef"=w715) -> ()  [unwired: 7 in, 3 out]
                n371 = call-poly <vilib>:"WPI_SolenoidSet.vi"("Value"=WPI_SolenoidValue."Forward", "SolenoidDevRef"=w711) -> ()  [unwired: 8 in, 2 out]
                n372 = call-poly <vilib>:"WPI_SolenoidSet.vi"("Value"=WPI_SolenoidValue."Reverse", "SolenoidDevRef"=w713) -> ()  [unwired: 8 in, 2 out]
              }
              frame "Approach Bar" {
                w716 = TRUE ("Climb Started?")
                # "Flip"
                # "Extend Pull-Up"
                # "Deploy climb \nmechanism"
                # "Approaches the bar and aligns. Deploys climb mechanism"
                # "Deploy Climb     Put elevator at 20 degrees     wait for driver command to continue"
                n373 = shared-variable ".\\Shared Variables.lvlib\\Ascent.lvlib\\Climb Started"(w716) -> ()  [unwired: 1 in, 1 out]
                n374 = call <vilib>:"WPI_EncoderGet.vi"("EncoderDevRef"=w726) -> ("Distance"=w722:dbl)  [unwired: 5 in, 5 out]
                n375 = Less Or Equal?(x=w722, y="distance to flip 2") -> (x <= y?=w721:bool)
                n376 = Select(t=climb_step_state."Approach +" ("Climb Step"), s=w721, f=climb_step_state."Approach Bar" ("Climb Step")) -> (s? t:f=w718:T1)
                n377 = Select(t=0.0, s=w721, f="Auto Flip Speed 2") -> (s? t:f=w723:dbl)
                n378 = call <vilib>:"WPI_MotorControlSetOutput.vi"("Output"=w723, "MotorControlDevRef"=w727) -> ()  [unwired: 7 in, 3 out]
                n379 = call-poly <vilib>:"WPI_SolenoidSet.vi"("Value"=WPI_SolenoidValue."Forward", "SolenoidDevRef"=w730) -> ()  [unwired: 8 in, 2 out]
                "Rung counter 3" <- 1 ("Rung counter")
                "Climb Started? 2" <- w716
              }
              frame "Approach +" {
                n380 = call <vilib>:"WPI_EncoderGet.vi"("EncoderDevRef"=w733) -> ("Distance"=w736:dbl)  [unwired: 5 in, 5 out]
                n381 = Greater Or Equal?(x=w736, y="half extend distance 2") -> (x >= y?=w738:bool)
                n382 = Select(t=climb_step_state."Check Continue" ("Climb Step"), s=w738, f=climb_step_state."Approach +" ("Climb Step")) -> (s? t:f=w731:T1)
                n383 = Select(t=0.0, s=w738, f=w732) -> (s? t:f=w739:dbl)
                n384 = call <vilib>:"WPI_MotorControlSetOutput.vi"("Output"=w739, "MotorControlDevRef"=w734) -> ()  [unwired: 7 in, 3 out]
              }
              frame "Climb Step 1" {
                # "Retract Pull-Up"
                # "Engage the pull up bars (lift robot off ground)"
                # "Do a pullup"
                n385 = call-poly <vilib>:"WPI_SolenoidSet.vi"("Value"=WPI_SolenoidValue."Reverse", "SolenoidDevRef"=w744) -> ()  [unwired: 8 in, 2 out]
              }
              frame "Climb Step 2" {
                # "Extending the tail hook to a wanted distance. Runs until distance is reached"
                # "Extend tail hook a given amount"
                n386 = local read "Disciplined Sky Enc 2"() -> (w746:dbl)
                n387 = Greater Or Equal?(x=w746, y="distance to extend 3") -> (x >= y?=w745:bool)
                n388 = Select(t=climb_step_state."Climb Step 2" ("Climb Step"), s=w745, f=w748) -> (s? t:f=w750:T1)
                n389 = Select(t=0.0, s=w745, f=w747) -> (s? t:f=w752:dbl)
                n390 = call <vilib>:"WPI_MotorControlSetOutput.vi"("Output"=w752, "MotorControlDevRef"=w751) -> ()  [unwired: 7 in, 3 out]
              }
              frame "Climb Step 3" {
                # "Engaging the slapper"
                # "Slap"
                n391 = call-poly <vilib>:"WPI_SolenoidSet.vi"("Value"=WPI_SolenoidValue."Forward", "SolenoidDevRef"=w757) -> ()  [unwired: 8 in, 2 out]
              }
              frame "Climb Step 4" {
                # "Retracting the tail hook enough to detect weight on sensor.\nRepeats until distance is reached."
                # "Start Retracting tail hook untill a given amount has been retracted"
                n392 = local read "Disciplined Sky Enc 2"() -> (w758:dbl)
                n393 = Greater Or Equal?(x=w758, y="Distance desired to \nretract (enough to detect if\nwe have weight on current sensor\nin next case) 3") -> (x >= y?=w763:bool)
                n394 = Select(t=climb_step_state."Climb Step 5" ("Climb Step"), s=w763, f=w760) -> (s? t:f=w762:T1)
                n395 = call <vilib>:"WPI_MotorControlSetOutput.vi"("Output"=-1.0 ("f"), "MotorControlDevRef"=w765) -> ()  [unwired: 7 in, 3 out]
              }
              frame "Climb Step 5" {
                # "Check the load on current sensor. If false abort, if true\ngoes to next state"
                # "Check the current sensor abort if no current spike, else continue"
                n396 = call <vilib>:"WPI_AnalogChannelGetVoltage.vi"("AIDeviceRef"=w775) -> ("Voltage"=w774:dbl)  [unwired: 8 in, 2 out]
                n397 = Greater Or Equal?(x=w774, y="Current sensor load 3") -> (x >= y?=w772:bool)
                n398 = case shown="True" w772 {
                  selector: w772 -> [w776 w777]
                  tunnel: w771 -> [_ w781]
                  tunnel: w770 -> [_ w778]
                  tunnel: [w776 w777] -> w767
                  frame False {
                  }
                  frame True {
                    n399 = call-poly <vilib>:"WPI_SolenoidSet.vi"("Value"=WPI_SolenoidValue."Forward", "SolenoidDevRef"=w778) -> ()  [unwired: 8 in, 2 out]
                    n400 = call-poly <vilib>:"WPI_SolenoidSet.vi"("Value"=WPI_SolenoidValue."Reverse", "SolenoidDevRef"=w781) -> ()  [unwired: 8 in, 2 out]
                  }
                }
                n401 = Select(t=climb_step_state."Climb Step 6" ("Climb Step"), s=w767, f=climb_step_state."Abort" ("Climb Step")) -> (s? t:f=w769:T1)
              }
              frame "Climb Step 6" {
                # "Tail hook is retracted completely and pull up bar is engaged.\nWe are now hanging on rung 2 (if true). Repeats until true\nand then repeats process to climb to rung to in order to climb\nto rung 3"
                # "Once fully retracted do another pulluo"
                n402 = call <vilib>:"WPI_EncoderGet.vi"("EncoderDevRef"=w794) -> ()  [unwired: 5 in, 6 out]
                n403 = local read "Disciplined Sky Enc 2"() -> (w782:dbl)
                n404 = Greater Or Equal?(x=w782, y="Distance desired to\nretract tail hook completely 3") -> (x >= y?=w789:bool)
                n405 = case shown="True" w789 {
                  selector: w789 -> [w795 w796]
                  tunnel: w788 -> [_ w797]
                  tunnel: [w795 w796] -> w787
                  frame False {
                  }
                  frame True {
                    n406 = call-poly <vilib>:"WPI_SolenoidSet.vi"("Value"=WPI_SolenoidValue."Reverse", "SolenoidDevRef"=w797) -> ()  [unwired: 8 in, 2 out]
                  }
                }
                n407 = Select(t=0.0, s=w789, f=w783) -> (s? t:f=w791:dbl)
                n408 = call <vilib>:"WPI_MotorControlSetOutput.vi"("Output"=w791, "MotorControlDevRef"=w790) -> ()  [unwired: 7 in, 3 out]
                n409 = Select(t=climb_step_state."Check Finished" ("Climb Step"), s=w787, f=w784) -> (s? t:f=w785:T1)
              }
              frame "Check Finished" {
                # "Rung counter keeps track of how many bars have been climbed.Once rung counter reaches 3\nit aborts the climb because it has finished. If less than 3 it will go back to case 2 to finish the climb"
                # "Check to see if we have climbed to level 3"
                n410 = local read "Rung counter 3"() -> (w805:i32)
                n411 = Increment(x=w805) -> (x+1=w799:i32)
                n412 = local write "Rung counter 3"(w799) -> ()
                n413 = Less?(x=w799, y=3) -> (x < y?=w803:bool)
                n414 = Select(t=climb_step_state."Check Continue" ("Climb Step"), s=w803, f=climb_step_state."Abort" ("Climb Step")) -> (s? t:f=w800:T1)
              }
              frame "Check Continue" {
                # "Get the go ahead from the driver to continue"
                n415 = shared-variable ".\\Shared Variables.lvlib\\Gamepad Driver.lvlib\\Dr Button 1"() -> (w806:bool)  [unwired: 1 in, 1 out]
                n416 = Not Equal?(x=w811, y=w807) -> (x != y?=w810:bool)
                n417 = feedback #15() -> (w809:T1)  [unwired: 1 in]
                n418 = case shown="True" w810 {
                  tunnel: w809 -> [w816 _]
                  tunnel: [w816 w817] -> w808
                  tunnel: w807 -> [_ w817]
                  frame False {
                  }
                  frame True {
                  }
                }
                n419 = feedback-in #15(w808) -> ()
                n420 = feedback #16(FALSE ("Button 1")) -> (w815:bool)
                n421 = feedback-in #16(w806) -> ()
                n422 = Greater?(x=w806, y=w815) -> (0:w813:bool)
                n423 = case shown="\"Check Finished\"" w808 {
                  selector: w808 -> [w818 _ _ w829 w832]
                  tunnel: w813 -> [_ w822 w826 w828 w833]
                  tunnel: [w818 w820 w823 w827 w831] -> w812
                  tunnel: w811 -> [_ w819 w825 _ _]
                  frame "Abort", Default {
                    # "This is a final case once here you are done in automatic mode"
                  }
                  frame "Approach Bar" {
                    # "This Case not exercised in Check Continue,\nsince Approach + happens immediately after Approach Bar"
                    # "The climb mechinism is now folded out, and we are awaiting the \ndriver to tell us that its ok to do the first chin up ie 10 point climb"
                    n424 = Select(t=climb_step_state."Climb Step 1" ("Climb Step"), s=w822, f=w819) -> (s? t:f=w820:T1)
                  }
                  frame "Approach +" {
                    n425 = Select(t=climb_step_state."Climb Step 1" ("Climb Step"), s=w826, f=w825) -> (s? t:f=w823:T1)
                  }
                  frame "Climb Step 1" {
                    # "We are hanging off the first rung should we attempt the second"
                    n426 = Select(t=climb_step_state."Climb Step 2" ("Climb Step"), s=w828, f=w829) -> (s? t:f=w827:T1)
                  }
                  frame "Check Finished" {
                    # "We have climbed to the second rung should we go for the third ?\nIf os wrap back around and repeat the previous steps."
                    n427 = Select(t=climb_step_state."Climb Step 2" ("Climb Step"), s=w833, f=w832) -> (s? t:f=w831:T1)
                  }
                }
              }
            }
          }
          frame 3 {
          }
          frame 0, Default {
            # "Flip"
            n428 = call <vilib>:"WPI_ServoRefNum Registry Get.vi"("refnum name"="breakServo") -> ("ServoDeviceRef"=w837:T38)  [unwired: 9 in, 1 out]
            n429 = call <vilib>:"WPI_EncoderGet.vi"("EncoderDevRef"=w841) -> ("Distance"=→"Distance 2":dbl)  [unwired: 5 in, 5 out]
            n430 = call <vilib>:"WPI_ServoSetAngle.vi"("Angle"=0, "ServoDeviceRef"=w837) -> ()  [unwired: 8 in, 2 out]
            n431 = call <vilib>:"WPI_MotorControlSetOutput.vi"("Output"="Output 2", "MotorControlDevRef"=w840) -> ()  [unwired: 7 in, 3 out]
          }
          frame 2 {
            # "Only can manually \nclimb after climb has\nbeen activated"
            n432 = shared-variable ".\\Shared Variables.lvlib\\Ascent.lvlib\\Climb Started"() -> (w844:bool)  [unwired: 1 in, 1 out]
            n433 = case shown="True" w844 {
              tunnel: w853 -> [_ w877]
              tunnel: w852 -> [_ w874]
              tunnel: w851 -> [_ _]
              tunnel: w849 -> [_ w863]
              tunnel: w848 -> [_ w865]
              tunnel: w847 -> [_ w864]
              tunnel: w846 -> [_ w862]
              tunnel: w845 -> [_ w861]
              frame False {
              }
              frame True {
                # "Slow Retract"
                # "Slow Extend"
                # "Climb Extend Tail Speed"
                # "Climb Retract Tail Speed"
                # "Man Flip Speed"
                # "Slow"
                # "Extend"
                # "Retract"
                # "Slapper"
                # "Pull Up"
                n434 = shared-variable ".\\Shared Variables.lvlib\\Ascent.lvlib\\Slapper State"() -> (w855:bool)  [unwired: 1 in, 1 out]
                n435 = shared-variable ".\\Shared Variables.lvlib\\Ascent.lvlib\\ChinUp State"() -> (w854:bool)  [unwired: 1 in, 1 out]
                n436 = shared-variable ".\\Shared Variables.lvlib\\Gamepad Driver.lvlib\\Dr Button 5"() -> (w860:bool)  [unwired: 1 in, 1 out]
                n437 = shared-variable ".\\Shared Variables.lvlib\\Gamepad Driver.lvlib\\Dr Button 6"() -> (w859:bool)  [unwired: 1 in, 1 out]
                n438 = shared-variable ".\\Shared Variables.lvlib\\Gamepad Driver.lvlib\\Dr Button 7"() -> (w858:bool)  [unwired: 1 in, 1 out]
                n439 = case shown="False" w854 {
                  tunnel: [WPI_SolenoidValue."Reverse" ("Value") WPI_SolenoidValue."Forward" ("Value")] -> w875
                  frame False {
                  }
                  frame True {
                  }
                }
                n440 = case shown="False" w855 {
                  tunnel: [WPI_SolenoidValue."Reverse" ("Value") WPI_SolenoidValue."Forward" ("Value")] -> w876
                  frame False {
                  }
                  frame True {
                  }
                }
                n441 = call-poly <vilib>:"WPI_SolenoidSet.vi"("Value"=w875, "SolenoidDevRef"=w874) -> ()  [unwired: 8 in, 2 out]
                n442 = call-poly <vilib>:"WPI_SolenoidSet.vi"("Value"=w876, "SolenoidDevRef"=w877) -> ()  [unwired: 8 in, 2 out]
                n443 = feedback #17() -> (w869:dbl)  [unwired: 1 in]
                n444 = feedback #18(enum16{"Engaged", "Untension", "Disengaged"}."Disengaged") -> (w871:enum16{"Engaged", "Untension", "Disengaged"})
                n445 = call <vilib>:"WPI_ServoRefNum Registry Get.vi"("refnum name"="breakServo") -> ("ServoDeviceRef"=w866:T38)  [unwired: 9 in, 1 out]
                n446 = case shown="\"Untension\"" w871 {
                  tunnel: [w889 w912 w925] -> w867
                  tunnel: ["Motor Pwr 2" w906 w922] -> w856
                  tunnel: [w880 w904 w921] -> w870
                  tunnel: w869 -> [w880 _ w921]
                  tunnel: w866 -> [w883 w900 _]
                  tunnel: w860 -> [_ w898 w914]
                  tunnel: w859 -> [_ w897 w916]
                  tunnel: w865 -> [_ w896 _]
                  tunnel: w864 -> [_ _ _]
                  tunnel: w858 -> [_ w895 w917]
                  tunnel: w863 -> [_ _ w918]
                  tunnel: w862 -> [_ _ w913]
                  tunnel: w861 -> [_ w894 _]
                  frame "Untension" {
                    # "Moves the motor backwards for a certain time then switches to the disengage"
                    n447 = Get Date/Time In Seconds() -> (seconds since 1Jan1904=w891:timestamp)
                    n448 = Add(x="Delay for disengage 2", y=w880) -> (x+y=w882:dbl)
                    n449 = To Double Precision Float(number=w891) -> (double precision float=w881:dbl)
                    n450 = Add(x="Motor Run Time 2", y=w880) -> (x+y=w888:dbl)
                    n451 = Greater?(x=w881, y=w882) -> (0:w878:bool)
                    n452 = Greater?(x=w881, y=w888) -> (0:w890:bool)
                    n453 = Select(t=enum16{"Engaged", "Untension", "Disengaged"}."Disengaged", s=w890, f=enum16{"Engaged", "Untension", "Disengaged"}."Untension") -> (s? t:f=w889:enum16{"Engaged", "Untension", "Disengaged"})
                    n454 = case shown="True" w878 {
                      tunnel: w883 -> [_ w892]
                      frame False {
                      }
                      frame True {
                        n455 = call <vilib>:"WPI_ServoSetAngle.vi"("Angle"="Break Disengaged 2", "ServoDeviceRef"=w892) -> ()  [unwired: 8 in, 2 out]
                      }
                    }
                  }
                  frame "Engaged" {
                    # "button 5 switches the case to untension\nbutton 6 retracts without changing state\nengages the break, cant extend\notherwise stay in this case."
                    # "Rising Edge"
                    n456 = feedback-in #19(w898) -> ()
                    n457 = feedback #19() -> (w899:bool)  [unwired: 1 in]
                    n458 = Greater?(x=w898, y=w899) -> (0:w910:bool)
                    n459 = Get Date/Time In Seconds() -> (seconds since 1Jan1904=w905:timestamp)
                    n460 = Select(t=enum16{"Engaged", "Untension", "Disengaged"}."Untension", s=w910, f=enum16{"Engaged", "Untension", "Disengaged"}."Engaged") -> (s? t:f=w912:enum16{"Engaged", "Untension", "Disengaged"})
                    n461 = To Double Precision Float(number=w905) -> (double precision float=w904:dbl)
                    n462 = Not(x=w897) -> (.not. x?=w911:bool)
                    n463 = Or(x=w910, y=w911) -> (x .or. y?=w908:bool)
                    n464 = Select(t=w894, s=w895, f=w896) -> (s? t:f=w909:dbl)
                    n465 = Select(t=0, s=w908, f=w909) -> (s? t:f=w906:dbl)
                    n466 = call <vilib>:"WPI_ServoSetAngle.vi"("Angle"="Break Engaged 2", "ServoDeviceRef"=w900) -> ()  [unwired: 8 in, 2 out]
                  }
                  frame "Disengaged" {
                    # "Button 6  retacts the skyhook and is supposed to change the state to engaged and engage the break\nbutton 5 extends the skyhook\ndisengages the break, free to extend\notherwise stay in this case"
                    n467 = feedback-in #20(w916) -> ()
                    n468 = feedback #20() -> (w915:bool)  [unwired: 1 in]
                    n469 = Greater?(x=w916, y=w915) -> (0:w926:bool)
                    n470 = Select(t=enum16{"Engaged", "Untension", "Disengaged"}."Engaged", s=w926, f=enum16{"Engaged", "Untension", "Disengaged"}."Disengaged") -> (s? t:f=w925:enum16{"Engaged", "Untension", "Disengaged"})
                    n471 = Select(t=w913, s=w917, f=w918) -> (s? t:f=w924:dbl)
                    n472 = Select(t=w924, s=w914, f=0) -> (s? t:f=w922:dbl)
                  }
                }
                "Enum 2" <- w867
                n473 = feedback-in #17(w870) -> ()
                n474 = feedback-in #18(w867) -> ()
                n475 = call <vilib>:"WPI_MotorControlRefNum Registry Get.vi"("refnum name"="climbMotor") -> ("MotorControlDevRef"=w857:T8)  [unwired: 9 in, 1 out]
                n476 = call "SimpleSetMotor.vi"("Output"=w856, "MotorControlDevRef"=w857) -> ()  [unwired: 8 in, 2 out]
              }
            }
          }
        }
        n477 = feedback #21(0.0) -> (w670:dbl)
        n478 = case shown="True" w666 {
          tunnel: w667 -> [_ w692]
          tunnel: [w690 w691] -> w668
          tunnel: w670 -> [w690 _]
          frame False {
          }
          frame True {
            n479 = Subtract(x="Sky Home Position 2", y=w692) -> (x-y=w691:dbl)
            "Turret Home Adjust 2" <- w691
          }
        }
        n480 = feedback-in #21(w668) -> ()
        n481 = Add(x=w667, y=w668) -> (x+y=w662:dbl)
        "Disciplined Sky Enc 2" <- w662
        n482 = call <vilib>:"SD Write Number.vi"("Numeric"=w662, "Name"="climbEncoder_i") -> ()  [unwired: 8 in, 2 out]
        n483 = Wait (ms)(milliseconds to wait=u32 50) -> ()  [unwired: 1 out]
        "Climb Step 2" <- w681
      }
    }
    frame Enabled {
    }
  }
